vi "myRIO_BRig_Host_endExp_storeFiles__v3.vi"(0 "input_filePath":path) -> ()   [LabVIEW 2014]
panel:
  out "error2":errorcluster
  out "error1":errorcluster
  in  "input_error":errorcluster
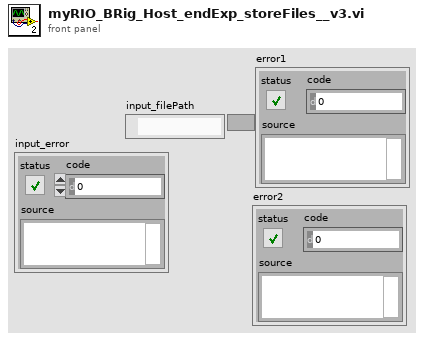
[diagram p1: front panel]
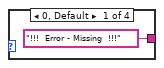
[diagram p2: hidden frame]
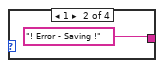
[diagram p3: hidden frame]
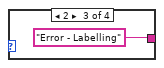
[diagram p4: hidden frame]
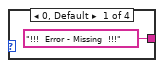
[diagram p5: hidden frame]
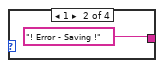
[diagram p6: hidden frame]
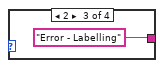
[diagram p7: hidden frame]
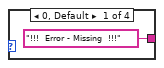
[diagram p8: hidden frame]
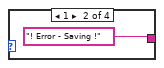
[diagram p9: hidden frame]
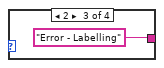
[diagram p10: hidden frame]
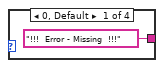
[diagram p11: hidden frame]
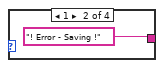
[diagram p12: hidden frame]
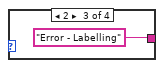
[diagram p13: hidden frame]
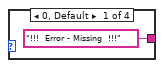
[diagram p14: hidden frame]
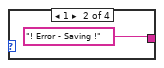
[diagram p15: hidden frame]
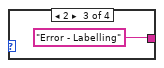
[diagram p16: hidden frame]
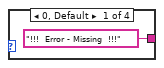
[diagram p17: hidden frame]
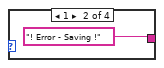
[diagram p18: hidden frame]
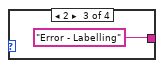
[diagram p19: hidden frame]
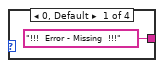
[diagram p20: hidden frame]
diagram:
  w2 = "\r"
  # "Workbooks"
  # "Application"
  # "Is Excel Running?"
  n1 = flat-sequence {
    tunnel: "input_filePath" -> [w358]
    tunnel: "input_error" -> [w355]
    tunnel: [w354] -> w350
    tunnel: [w357] -> w349
    tunnel: [w356] -> w348
    tunnel: [w353] -> w346
    tunnel: w350 -> [w396]
    tunnel: w349 -> [w397]
    tunnel: w348 -> [w360]
    tunnel: [w397] -> w347
    tunnel: w346 -> [w359]
    tunnel: [w396] -> w345
    tunnel: [w392] -> w344
    tunnel: [w391] -> w343
    tunnel: [w387] -> w269
    tunnel: [w386] -> w262
    tunnel: [w383] -> w234
    tunnel: [w380] -> w233
    tunnel: [w379] -> w232
    tunnel: [w378] -> w231
    tunnel: [w372] -> w223
    tunnel: [w371] -> w222
    tunnel: [w367] -> w221
    tunnel: [w366] -> w220
    tunnel: [w362] -> w219
    tunnel: [w361] -> w218
    tunnel: w347 -> [w434]
    tunnel: w345 -> [w430]
    tunnel: w344 -> [w429]
    tunnel: w343 -> [w433]
    tunnel: [w434] -> w342
    tunnel: [w432] -> w341
    tunnel: [w431] -> w340
    tunnel: [w403] -> w339
    tunnel: [w429] -> w338
    tunnel: [w428] -> w270
    tunnel: w269 -> [w428]
    tunnel: [w426] -> w263
    tunnel: w262 -> [w427]
    tunnel: [w425] -> w261
    tunnel: w234 -> [w423]
    tunnel: w233 -> [w422]
    tunnel: w232 -> [w410]
    tunnel: w231 -> [w412]
    tunnel: [w423] -> w225
    tunnel: w223 -> [w421]
    tunnel: w222 -> [w414]
    tunnel: w221 -> [w420]
    tunnel: w220 -> [w416]
    tunnel: w219 -> [w419]
    tunnel: w218 -> [w418]
    tunnel: [w409] -> w212
    tunnel: [w422] -> w206
    tunnel: [w411] -> w200
    tunnel: [w421] -> w194
    tunnel: [w413] -> w188
    tunnel: [w420] -> w182
    tunnel: [w415] -> w176
    tunnel: [w419] -> w170
    tunnel: [w417] -> w164
    tunnel: [w402] -> w163
    tunnel: [w401] -> w153
    tunnel: [w400] -> w145
    tunnel: [w399] -> w139
    tunnel: [w398] -> w134
    tunnel: w342 -> [w471]
    tunnel: w341 -> [w469]
    tunnel: w340 -> [w468]
    tunnel: w339 -> [w443]
    tunnel: w338 -> [w470]
    tunnel: [w471] -> w325
    tunnel: [w470] -> w323
    tunnel: [w469] -> w321
    tunnel: [w468] -> w319
    tunnel: [w467] -> w317
    tunnel: [w462] -> w315
    tunnel: [w464] -> w271
    tunnel: w270 -> [w464]
    tunnel: [w465] -> w264
    tunnel: w263 -> [w465]
    tunnel: w261 -> [w466]
    tunnel: [w466] -> w260
    tunnel: [w463] -> w256
    tunnel: [w459] -> w226
    tunnel: w225 -> [w459]
    tunnel: [w460] -> w213
    tunnel: w212 -> [w460]
    tunnel: [w455] -> w207
    tunnel: w206 -> [w455]
    tunnel: [w456] -> w201
    tunnel: w200 -> [w456]
    tunnel: [w446] -> w195
    tunnel: w194 -> [w446]
    tunnel: [w449] -> w189
    tunnel: w188 -> [w449]
    tunnel: [w445] -> w183
    tunnel: w182 -> [w445]
    tunnel: [w448] -> w177
    tunnel: w176 -> [w448]
    tunnel: [w444] -> w171
    tunnel: w170 -> [w444]
    tunnel: [w447] -> w165
    tunnel: w164 -> [w447]
    tunnel: w163 -> [w461]
    tunnel: [w461] -> w159
    tunnel: [w458] -> w158
    tunnel: w153 -> [w457]
    tunnel: [w457] -> w151
    tunnel: [w454] -> w148
    tunnel: [w453] -> w146
    tunnel: w145 -> [w450]
    tunnel: [w450] -> w140
    tunnel: w139 -> [w451]
    tunnel: [w451] -> w135
    tunnel: w134 -> [w452]
    tunnel: [w452] -> w130
    tunnel: [w442] -> w129
    tunnel: [w441] -> w124
    tunnel: [w440] -> w119
    tunnel: [w439] -> w110
    tunnel: [w438] -> w108
    tunnel: [w437] -> w106
    tunnel: [w436] -> w104
    tunnel: [w435] -> w102
    tunnel: w325 -> [w566]
    tunnel: [w566] -> w324
    tunnel: w323 -> [w565]
    tunnel: [w565] -> w322
    tunnel: w321 -> [w564]
    tunnel: [w564] -> w320
    tunnel: w319 -> [w563]
    tunnel: [w563] -> w318
    tunnel: w317 -> [w561]
    tunnel: [w561] -> w316
    tunnel: w315 -> [w562]
    tunnel: [w562] -> w314
    tunnel: [w557] -> w272
    tunnel: w271 -> [w557]
    tunnel: [w556] -> w265
    tunnel: w264 -> [w556]
    tunnel: w260 -> [w555]
    tunnel: [w555] -> w259
    tunnel: w256 -> [w554]
    tunnel: [w554] -> w255
    tunnel: [w553] -> w227
    tunnel: w226 -> [w553]
    tunnel: [w552] -> w214
    tunnel: w213 -> [w552]
    tunnel: [w551] -> w208
    tunnel: w207 -> [w551]
    tunnel: [w550] -> w202
    tunnel: w201 -> [w550]
    tunnel: [w549] -> w196
    tunnel: w195 -> [w549]
    tunnel: [w548] -> w190
    tunnel: w189 -> [w548]
    tunnel: [w547] -> w184
    tunnel: w183 -> [w547]
    tunnel: [w546] -> w178
    tunnel: w177 -> [w546]
    tunnel: [w545] -> w172
    tunnel: w171 -> [w545]
    tunnel: [w544] -> w166
    tunnel: w165 -> [w544]
    tunnel: [w543] -> w160
    tunnel: w159 -> [w543]
    tunnel: w158 -> [w542]
    tunnel: [w542] -> w154
    tunnel: [w541] -> w152
    tunnel: w151 -> [w541]
    tunnel: w148 -> [w533]
    tunnel: [w540] -> w147
    tunnel: w146 -> [w540]
    tunnel: [w539] -> w141
    tunnel: w140 -> [w539]
    tunnel: [w538] -> w136
    tunnel: w135 -> [w538]
    tunnel: [w537] -> w131
    tunnel: w130 -> [w537]
    tunnel: w129 -> [w536]
    tunnel: [w536] -> w125
    tunnel: w124 -> [w535]
    tunnel: [w535] -> w120
    tunnel: w119 -> [w534]
    tunnel: [w534] -> w115
    tunnel: [w533] -> w111
    tunnel: w110 -> [w532]
    tunnel: [w532] -> w109
    tunnel: w108 -> [w531]
    tunnel: [w531] -> w107
    tunnel: w106 -> [w530]
    tunnel: [w530] -> w105
    tunnel: w104 -> [w529]
    tunnel: [w529] -> w103
    tunnel: w102 -> [w528]
    tunnel: [w528] -> w101
    tunnel: w324 -> [w623]
    tunnel: w322 -> [w622]
    tunnel: w320 -> [w620]
    tunnel: w318 -> [w619]
    tunnel: w316 -> [w621]
    tunnel: w314 -> [w616]
    tunnel: [w623] -> w337
    tunnel: [w622] -> w336
    tunnel: [w621] -> w335
    tunnel: [w603] -> w334
    tunnel: [w618] -> w333
    tunnel: [w617] -> w332
    tunnel: [w615] -> w273
    tunnel: w272 -> [w615]
    tunnel: [w611] -> w266
    tunnel: w265 -> [w613]
    tunnel: w259 -> [w612]
    tunnel: w255 -> [w614]
    tunnel: [w614] -> w254
    tunnel: [w610] -> w251
    tunnel: [w609] -> w228
    tunnel: w227 -> [w609]
    tunnel: [w570] -> w215
    tunnel: w214 -> [w596]
    tunnel: [w608] -> w209
    tunnel: w208 -> [w608]
    tunnel: [w573] -> w203
    tunnel: w202 -> [w593]
    tunnel: [w607] -> w197
    tunnel: w196 -> [w607]
    tunnel: [w576] -> w191
    tunnel: w190 -> [w590]
    tunnel: [w606] -> w185
    tunnel: w184 -> [w606]
    tunnel: [w579] -> w179
    tunnel: w178 -> [w587]
    tunnel: [w605] -> w173
    tunnel: w172 -> [w605]
    tunnel: [w582] -> w167
    tunnel: w166 -> [w597]
    tunnel: w160 -> [w595]
    tunnel: [w604] -> w155
    tunnel: w154 -> [w604]
    tunnel: w152 -> [w592]
    tunnel: w147 -> [w602]
    tunnel: [w581] -> w142
    tunnel: w141 -> [w584]
    tunnel: w136 -> [w586]
    tunnel: w131 -> [w589]
    tunnel: [w601] -> w126
    tunnel: w125 -> [w601]
    tunnel: [w600] -> w121
    tunnel: w120 -> [w600]
    tunnel: [w599] -> w116
    tunnel: w115 -> [w599]
    tunnel: [w598] -> w112
    tunnel: w111 -> [w598]
    tunnel: w109 -> [w594]
    tunnel: w107 -> [w591]
    tunnel: w105 -> [w588]
    tunnel: w103 -> [w585]
    tunnel: w101 -> [w583]
    tunnel: [w580] -> w100
    tunnel: [w578] -> w99
    tunnel: [w577] -> w98
    tunnel: [w575] -> w97
    tunnel: [w574] -> w96
    tunnel: [w572] -> w95
    tunnel: [w571] -> w94
    tunnel: [w569] -> w93
    tunnel: [w568] -> w92
    tunnel: [w567] -> w91
    tunnel: w337 -> [w743]
    tunnel: w336 -> [w741]
    tunnel: w335 -> [w735]
    tunnel: w334 -> [w739]
    tunnel: w333 -> [w742]
    tunnel: w332 -> [w737]
    tunnel: [w743] -> w331
    tunnel: [w741] -> w330
    tunnel: [w740] -> w329
    tunnel: [w727] -> w328
    tunnel: [w742] -> w327
    tunnel: [w737] -> w326
    tunnel: [w733] -> w274
    tunnel: w273 -> [w733]
    tunnel: [w732] -> w267
    tunnel: w266 -> [w732]
    tunnel: [w728] -> w258
    tunnel: w254 -> [w730]
    tunnel: [w729] -> w253
    tunnel: w251 -> [w728]
    tunnel: [w718] -> w229
    tunnel: w228 -> [w718]
    tunnel: [w719] -> w216
    tunnel: w215 -> [w719]
    tunnel: [w711] -> w210
    tunnel: w209 -> [w711]
    tunnel: [w712] -> w204
    tunnel: w203 -> [w712]
    tunnel: [w703] -> w198
    tunnel: w197 -> [w703]
    tunnel: [w704] -> w192
    tunnel: w191 -> [w704]
    tunnel: [w690] -> w186
    tunnel: w185 -> [w690]
    tunnel: [w691] -> w180
    tunnel: w179 -> [w691]
    tunnel: [w684] -> w174
    tunnel: w173 -> [w684]
    tunnel: [w685] -> w168
    tunnel: w167 -> [w685]
    tunnel: [w721] -> w161
    tunnel: [w723] -> w156
    tunnel: w155 -> [w724]
    tunnel: [w715] -> w149
    tunnel: [w692] -> w143
    tunnel: w142 -> [w692]
    tunnel: [w693] -> w137
    tunnel: [w694] -> w132
    tunnel: [w680] -> w127
    tunnel: w126 -> [w682]
    tunnel: [w687] -> w122
    tunnel: w121 -> [w686]
    tunnel: [w700] -> w117
    tunnel: w116 -> [w701]
    tunnel: [w709] -> w113
    tunnel: w112 -> [w708]
    tunnel: w100 -> [w683]
    tunnel: w99 -> [w693]
    tunnel: w98 -> [w689]
    tunnel: w97 -> [w694]
    tunnel: w96 -> [w702]
    tunnel: w95 -> [w715]
    tunnel: w94 -> [w710]
    tunnel: w93 -> [w721]
    tunnel: w92 -> [w717]
    tunnel: w91 -> [w726]
    tunnel: [w725] -> w89
    tunnel: [w716] -> w87
    tunnel: [w707] -> w85
    tunnel: [w699] -> w83
    tunnel: [w688] -> w81
    tunnel: [w681] -> w79
    tunnel: w331 -> [w830]
    tunnel: w330 -> [w835]
    tunnel: w329 -> [w834]
    tunnel: w328 -> [w833]
    tunnel: w327 -> [w832]
    tunnel: w326 -> [w831]
    tunnel: [w830] -> w313
    tunnel: [w835] -> w312
    tunnel: [w834] -> w311
    tunnel: [w833] -> w310
    tunnel: [w832] -> w309
    tunnel: [w831] -> w308
    tunnel: [w829] -> w275
    tunnel: w274 -> [w829]
    tunnel: [w828] -> w268
    tunnel: w267 -> [w828]
    tunnel: w258 -> [w827]
    tunnel: [w827] -> w257
    tunnel: w253 -> [w826]
    tunnel: [w826] -> w252
    tunnel: [w825] -> w230
    tunnel: w229 -> [w825]
    tunnel: [w824] -> w217
    tunnel: w216 -> [w824]
    tunnel: [w823] -> w211
    tunnel: w210 -> [w823]
    tunnel: [w822] -> w205
    tunnel: w204 -> [w822]
    tunnel: [w821] -> w199
    tunnel: w198 -> [w821]
    tunnel: [w820] -> w193
    tunnel: w192 -> [w820]
    tunnel: [w819] -> w187
    tunnel: w186 -> [w819]
    tunnel: [w818] -> w181
    tunnel: w180 -> [w818]
    tunnel: [w817] -> w175
    tunnel: w174 -> [w817]
    tunnel: [w816] -> w169
    tunnel: w168 -> [w816]
    tunnel: [w815] -> w162
    tunnel: w161 -> [w815]
    tunnel: [w814] -> w157
    tunnel: w156 -> [w814]
    tunnel: [w813] -> w150
    tunnel: w149 -> [w813]
    tunnel: [w812] -> w144
    tunnel: w143 -> [w812]
    tunnel: [w811] -> w138
    tunnel: w137 -> [w811]
    tunnel: [w810] -> w133
    tunnel: w132 -> [w810]
    tunnel: [w809] -> w128
    tunnel: w127 -> [w809]
    tunnel: [w808] -> w123
    tunnel: w122 -> [w808]
    tunnel: [w807] -> w118
    tunnel: w117 -> [w807]
    tunnel: [w806] -> w114
    tunnel: w113 -> [w806]
    tunnel: [w805] -> w90
    tunnel: w89 -> [w805]
    tunnel: [w804] -> w88
    tunnel: w87 -> [w804]
    tunnel: [w803] -> w86
    tunnel: w85 -> [w803]
    tunnel: [w802] -> w84
    tunnel: w83 -> [w802]
    tunnel: [w801] -> w82
    tunnel: w81 -> [w801]
    tunnel: [w800] -> w80
    tunnel: w79 -> [w800]
    tunnel: w313 -> [w874]
    tunnel: w312 -> [w882]
    tunnel: w311 -> [w881]
    tunnel: w310 -> [w880]
    tunnel: w309 -> [w879]
    tunnel: w308 -> [w878]
    tunnel: [w874] -> w305
    tunnel: [w882] -> w301
    tunnel: [w881] -> w300
    tunnel: [w880] -> w297
    tunnel: [w879] -> w299
    tunnel: [w878] -> w298
    tunnel: [w870] -> w304
    tunnel: [w869] -> w303
    tunnel: [w868] -> w302
    tunnel: [w867] -> w250
    tunnel: w275 -> [w867]
    tunnel: [w866] -> w248
    tunnel: w268 -> [w866]
    tunnel: w257 -> [w865]
    tunnel: [w865] -> w247
    tunnel: w252 -> [w864]
    tunnel: [w864] -> w249
    tunnel: [w863] -> w224
    tunnel: w230 -> [w863]
    tunnel: [w862] -> w77
    tunnel: w217 -> [w862]
    tunnel: [w861] -> w75
    tunnel: w211 -> [w861]
    tunnel: [w860] -> w73
    tunnel: w205 -> [w860]
    tunnel: [w859] -> w71
    tunnel: w199 -> [w859]
    tunnel: [w858] -> w69
    tunnel: w193 -> [w858]
    tunnel: [w857] -> w67
    tunnel: w187 -> [w857]
    tunnel: [w856] -> w65
    tunnel: w181 -> [w856]
    tunnel: [w855] -> w63
    tunnel: w175 -> [w855]
    tunnel: [w854] -> w61
    tunnel: w169 -> [w854]
    tunnel: [w853] -> w76
    tunnel: w162 -> [w853]
    tunnel: [w852] -> w78
    tunnel: w157 -> [w852]
    tunnel: [w851] -> w72
    tunnel: w150 -> [w851]
    tunnel: [w850] -> w60
    tunnel: w144 -> [w850]
    tunnel: [w849] -> w64
    tunnel: w138 -> [w849]
    tunnel: [w848] -> w68
    tunnel: w133 -> [w848]
    tunnel: [w847] -> w62
    tunnel: w128 -> [w847]
    tunnel: [w846] -> w66
    tunnel: w123 -> [w846]
    tunnel: [w845] -> w70
    tunnel: w118 -> [w845]
    tunnel: [w844] -> w74
    tunnel: w114 -> [w844]
    tunnel: [w843] -> w59
    tunnel: w90 -> [w843]
    tunnel: [w842] -> w58
    tunnel: w88 -> [w842]
    tunnel: [w841] -> w57
    tunnel: w86 -> [w841]
    tunnel: [w840] -> w56
    tunnel: w84 -> [w840]
    tunnel: [w839] -> w55
    tunnel: w82 -> [w839]
    tunnel: [w838] -> w54
    tunnel: w80 -> [w838]
    frame #0 {
      # "Is Excel Running?"
      # "Prepare storage"
      # "get Exp Prefix"
      n2 = call "myRIO_BRig_Host_endExp_getExp.vi"("input_filePath"=w358) -> ("output_expPrefix"=w356:string)  [unwired: 10 in]
      n3 = call "myRIO_BRig_Host_isExcelRunning.vi"() -> ("output_Iexcel"=w357:bool)  [unwired: 11 in]
      n4 = call "myRIO_BRig_Host_endExp_prepareStoreLocation.vi"("input_error"=w355, "input_expPrefix"=w356) -> ("output_error"=w354:errorcluster, "output_folderPath"=w353:string)  [unwired: 8 in]
    }
    frame #1 {
      w363 = "dataTrial" ("input_fileName")
      w368 = "dataMTrig" ("input_fileName")
      w373 = "dataLick" ("input_fileName")
      w377 = "dataLC" ("input_fileName")
      w376 = "dataExp" ("input_fileName")
      w388 = "dataCurrent" ("input_fileName")
      w395 = "dataBlock" ("input_fileName")
      # "original"
      # "storage"
      # "original"
      # "storage"
      # "original"
      # "storage"
      # "original"
      # "storage"
      # "original"
      # "storage"
      # "original"
      # "storage"
      # "original"
      # "storage"
      # "Prepare file paths"
      n5 = call "myRIO_BRig_Host_endExp_filePath__originalLocation.vi"("input_expPrefix"=w360, "input_fileName"=w376) -> ("output_filePath"=w384:string)  [unwired: 9 in]
      n6 = call "myRIO_BRig_Host_endExp_filePath__storeLocation.vi"("input_expPrefix"=w360, "input_fileName"=w376, "input_filePath_storage"=w359) -> ("output_filePath"=w385:string)  [unwired: 8 in]
      n7 = call "myRIO_BRig_Host_endExp_filePath__originalLocation.vi"("input_expPrefix"=w360, "input_fileName"=w388) -> ("output_filePath"=w389:string)  [unwired: 9 in]
      n8 = call "myRIO_BRig_Host_endExp_filePath__originalLocation.vi"("input_expPrefix"=w360, "input_fileName"=w377) -> ("output_filePath"=w381:string)  [unwired: 9 in]
      n9 = call "myRIO_BRig_Host_endExp_filePath__originalLocation.vi"("input_expPrefix"=w360, "input_fileName"=w373) -> ("output_filePath"=w374:string)  [unwired: 9 in]
      n10 = call "myRIO_BRig_Host_endExp_filePath__originalLocation.vi"("input_expPrefix"=w360, "input_fileName"=w368) -> ("output_filePath"=w369:string)  [unwired: 9 in]
      n11 = call "myRIO_BRig_Host_endExp_filePath__originalLocation.vi"("input_expPrefix"=w360, "input_fileName"=w363) -> ("output_filePath"=w364:string)  [unwired: 9 in]
      n12 = call "myRIO_BRig_Host_endExp_filePath__storeLocation.vi"("input_expPrefix"=w360, "input_fileName"=w388, "input_filePath_storage"=w359) -> ("output_filePath"=w390:string)  [unwired: 8 in]
      n13 = call "myRIO_BRig_Host_endExp_filePath__storeLocation.vi"("input_expPrefix"=w360, "input_fileName"=w377, "input_filePath_storage"=w359) -> ("output_filePath"=w382:string)  [unwired: 8 in]
      n14 = call "myRIO_BRig_Host_endExp_filePath__storeLocation.vi"("input_expPrefix"=w360, "input_fileName"=w373, "input_filePath_storage"=w359) -> ("output_filePath"=w375:string)  [unwired: 8 in]
      n15 = call "myRIO_BRig_Host_endExp_filePath__storeLocation.vi"("input_expPrefix"=w360, "input_fileName"=w368, "input_filePath_storage"=w359) -> ("output_filePath"=w370:string)  [unwired: 8 in]
      n16 = call "myRIO_BRig_Host_endExp_filePath__storeLocation.vi"("input_expPrefix"=w360, "input_fileName"=w363, "input_filePath_storage"=w359) -> ("output_filePath"=w365:string)  [unwired: 8 in]
      n17 = call "myRIO_BRig_Host_endExp_filePath__originalLocation.vi"("input_expPrefix"=w360, "input_fileName"=w395) -> ("output_filePath"=w393:string)  [unwired: 9 in]
      n18 = call "myRIO_BRig_Host_endExp_filePath__storeLocation.vi"("input_expPrefix"=w360, "input_fileName"=w395, "input_filePath_storage"=w359) -> ("output_filePath"=w394:string)  [unwired: 8 in]
      n19 = String To Path(string=w385) -> (path=w383:path)
      n20 = String To Path(string=w384) -> (path=w379:path)
      n21 = String To Path(string=w390) -> (path=w387:path)
      n22 = String To Path(string=w389) -> (path=w386:path)
      n23 = String To Path(string=w382) -> (path=w380:path)
      n24 = String To Path(string=w381) -> (path=w378:path)
      n25 = String To Path(string=w375) -> (path=w372:path)
      n26 = String To Path(string=w374) -> (path=w371:path)
      n27 = String To Path(string=w370) -> (path=w367:path)
      n28 = String To Path(string=w369) -> (path=w366:path)
      n29 = String To Path(string=w365) -> (path=w362:path)
      n30 = String To Path(string=w364) -> (path=w361:path)
      n31 = String To Path(string=w394) -> (path=w392:path)
      n32 = String To Path(string=w393) -> (path=w391:path)
    }
    frame #2 {
      # "Check if\noriginal files\nexist"
      n33 = call "myRIO_BRig_generic_pathExists_fast_pathInput.vi"("input_error"=w430, "input_filePath"=w433) -> ("output_error"=w424:errorcluster, "output_Iexist"=w431:bool, "output_filePath"=w432:path)  [unwired: 7 in]
      n34 = call "myRIO_BRig_generic_pathExists_fast_pathInput.vi"("input_error"=w424, "input_filePath"=w427) -> ("output_error"=w408:errorcluster, "output_Iexist"=w425:bool, "output_filePath"=w426:path)  [unwired: 7 in]
      n35 = call "myRIO_BRig_generic_pathExists_fast_pathInput.vi"("input_error"=w408, "input_filePath"=w410) -> ("output_error"=w407:errorcluster, "output_Iexist"=w402:bool, "output_filePath"=w409:path)  [unwired: 7 in]
      n36 = call "myRIO_BRig_generic_pathExists_fast_pathInput.vi"("input_error"=w407, "input_filePath"=w412) -> ("output_error"=w406:errorcluster, "output_Iexist"=w401:bool, "output_filePath"=w411:path)  [unwired: 7 in]
      n37 = call "myRIO_BRig_generic_pathExists_fast_pathInput.vi"("input_error"=w406, "input_filePath"=w414) -> ("output_error"=w405:errorcluster, "output_Iexist"=w398:bool, "output_filePath"=w413:path)  [unwired: 7 in]
      n38 = call "myRIO_BRig_generic_pathExists_fast_pathInput.vi"("input_error"=w405, "input_filePath"=w416) -> ("output_error"=w404:errorcluster, "output_Iexist"=w399:bool, "output_filePath"=w415:path)  [unwired: 7 in]
      n39 = call "myRIO_BRig_generic_pathExists_fast_pathInput.vi"("input_error"=w404, "input_filePath"=w418) -> ("output_error"=w403:errorcluster, "output_Iexist"=w400:bool, "output_filePath"=w417:path)  [unwired: 7 in]
    }
    frame #3 {
      # "If original files exist,\nthen store them"
      n40 = case shown="True" w468 {
        selector: w468 -> [w520 w525]
        tunnel: w469 -> [_ w527]
        tunnel: w470 -> [_ w526]
        tunnel: w443 -> [w521 w524]
        tunnel: [w521 w523] -> w462
        tunnel: [w520 w522] -> w467
        frame False {
        }
        frame True {
          n41 = call "myRIO_BRig_generic_pathMove_pathInput.vi"("input_error"=w524, "input_Ioverwrite"=w525, "input_filePath_target"=w526, "input_filePath_source"=w527) -> ("output_error"=w523:errorcluster, "output_Iexist"=w522:bool)  [unwired: 5 in, 1 out]
        }
      }
      n42 = case shown="True" w466 {
        selector: w466 -> [w512 w517]
        tunnel: w465 -> [_ w519]
        tunnel: w464 -> [_ w518]
        tunnel: w443 -> [w513 w516]
        tunnel: [w513 w515] -> w453
        tunnel: [w512 w514] -> w463
        frame False {
        }
        frame True {
          n43 = call "myRIO_BRig_generic_pathMove_pathInput.vi"("input_error"=w516, "input_Ioverwrite"=w517, "input_filePath_target"=w518, "input_filePath_source"=w519) -> ("output_error"=w515:errorcluster, "output_Iexist"=w514:bool)  [unwired: 5 in, 1 out]
        }
      }
      n44 = case shown="True" w461 {
        selector: w461 -> [w504 w509]
        tunnel: w460 -> [_ w511]
        tunnel: w459 -> [_ w510]
        tunnel: w443 -> [w505 w508]
        tunnel: [w505 w507] -> w439
        tunnel: [w504 w506] -> w458
        frame False {
        }
        frame True {
          n45 = call "myRIO_BRig_generic_pathMove_pathInput.vi"("input_error"=w508, "input_Ioverwrite"=w509, "input_filePath_target"=w510, "input_filePath_source"=w511) -> ("output_error"=w507:errorcluster, "output_Iexist"=w506:bool)  [unwired: 5 in, 1 out]
        }
      }
      n46 = case shown="True" w457 {
        selector: w457 -> [w496 w501]
        tunnel: w456 -> [_ w503]
        tunnel: w455 -> [_ w502]
        tunnel: w443 -> [w497 w500]
        tunnel: [w497 w499] -> w438
        tunnel: [w496 w498] -> w454
        frame False {
        }
        frame True {
          n47 = call "myRIO_BRig_generic_pathMove_pathInput.vi"("input_error"=w500, "input_Ioverwrite"=w501, "input_filePath_target"=w502, "input_filePath_source"=w503) -> ("output_error"=w499:errorcluster, "output_Iexist"=w498:bool)  [unwired: 5 in, 1 out]
        }
      }
      n48 = case shown="True" w452 {
        selector: w452 -> [w488 w493]
        tunnel: w449 -> [_ w495]
        tunnel: w446 -> [_ w494]
        tunnel: w443 -> [w489 w492]
        tunnel: [w489 w491] -> w437
        tunnel: [w488 w490] -> w440
        frame False {
        }
        frame True {
          n49 = call "myRIO_BRig_generic_pathMove_pathInput.vi"("input_error"=w492, "input_Ioverwrite"=w493, "input_filePath_target"=w494, "input_filePath_source"=w495) -> ("output_error"=w491:errorcluster, "output_Iexist"=w490:bool)  [unwired: 5 in, 1 out]
        }
      }
      n50 = case shown="True" w451 {
        selector: w451 -> [w480 w485]
        tunnel: w448 -> [_ w487]
        tunnel: w445 -> [_ w486]
        tunnel: w443 -> [w481 w484]
        tunnel: [w481 w483] -> w436
        tunnel: [w480 w482] -> w441
        frame False {
        }
        frame True {
          n51 = call "myRIO_BRig_generic_pathMove_pathInput.vi"("input_error"=w484, "input_Ioverwrite"=w485, "input_filePath_target"=w486, "input_filePath_source"=w487) -> ("output_error"=w483:errorcluster, "output_Iexist"=w482:bool)  [unwired: 5 in, 1 out]
        }
      }
      n52 = case shown="True" w450 {
        selector: w450 -> [w472 w477]
        tunnel: w447 -> [_ w479]
        tunnel: w444 -> [_ w478]
        tunnel: w443 -> [w473 w476]
        tunnel: [w473 w475] -> w435
        tunnel: [w472 w474] -> w442
        frame False {
        }
        frame True {
          n53 = call "myRIO_BRig_generic_pathMove_pathInput.vi"("input_error"=w476, "input_Ioverwrite"=w477, "input_filePath_target"=w478, "input_filePath_source"=w479) -> ("output_error"=w475:errorcluster, "output_Iexist"=w474:bool)  [unwired: 5 in, 1 out]
        }
      }
    }
    frame #4 {
      # "Add a delay\nin case\nall files\nweren't stored"
      n54 = Select(t=u32 0 ("milliseconds to wait"), s=w561, f=u32 200 ("milliseconds to wait")) -> (s? t:f=w560:u32)
      n55 = Wait (ms)(milliseconds to wait=w560) -> ()  [unwired: 1 out]
    }
    frame #5 {
      # "Re-check\noriginal files"
      n56 = case shown="False" w619 {
        selector: w619 -> [_ w678]
        tunnel: w620 -> [w676 w679]
        tunnel: w616 -> [w675 w677]
        tunnel: [w674 w677] -> w603
        tunnel: [w673 w679] -> w618
        tunnel: [w672 w678] -> w617
        frame False {
          n57 = call "myRIO_BRig_generic_pathExists_fast_pathInput.vi"("input_error"=w675, "input_filePath"=w676) -> ("output_error"=w674:errorcluster, "output_Iexist"=w672:bool, "output_filePath"=w673:path)  [unwired: 7 in]
        }
        frame True {
        }
      }
      n58 = case shown="False" w612 {
        selector: w612 -> [_ w670]
        tunnel: w613 -> [w668 w671]
        tunnel: w602 -> [w667 w669]
        tunnel: [w666 w669] -> w567
        tunnel: [w665 w671] -> w611
        tunnel: [w664 w670] -> w610
        frame False {
          n59 = call "myRIO_BRig_generic_pathExists_fast_pathInput.vi"("input_error"=w667, "input_filePath"=w668) -> ("output_error"=w666:errorcluster, "output_Iexist"=w664:bool, "output_filePath"=w665:path)  [unwired: 7 in]
        }
        frame True {
        }
      }
      n60 = case shown="False" w595 {
        selector: w595 -> [_ w662]
        tunnel: w596 -> [w660 w663]
        tunnel: w594 -> [w659 w661]
        tunnel: [w658 w661] -> w568
        tunnel: [w657 w663] -> w570
        tunnel: [w656 w662] -> w569
        frame False {
          n61 = call "myRIO_BRig_generic_pathExists_fast_pathInput.vi"("input_error"=w659, "input_filePath"=w660) -> ("output_error"=w658:errorcluster, "output_Iexist"=w656:bool, "output_filePath"=w657:path)  [unwired: 7 in]
        }
        frame True {
        }
      }
      n62 = case shown="False" w592 {
        selector: w592 -> [_ w654]
        tunnel: w593 -> [w652 w655]
        tunnel: w591 -> [w651 w653]
        tunnel: [w650 w653] -> w571
        tunnel: [w649 w655] -> w573
        tunnel: [w648 w654] -> w572
        frame False {
          n63 = call "myRIO_BRig_generic_pathExists_fast_pathInput.vi"("input_error"=w651, "input_filePath"=w652) -> ("output_error"=w650:errorcluster, "output_Iexist"=w648:bool, "output_filePath"=w649:path)  [unwired: 7 in]
        }
        frame True {
        }
      }
      n64 = case shown="False" w589 {
        selector: w589 -> [_ w646]
        tunnel: w590 -> [w644 w647]
        tunnel: w588 -> [w643 w645]
        tunnel: [w642 w645] -> w574
        tunnel: [w641 w647] -> w576
        tunnel: [w640 w646] -> w575
        frame False {
          n65 = call "myRIO_BRig_generic_pathExists_fast_pathInput.vi"("input_error"=w643, "input_filePath"=w644) -> ("output_error"=w642:errorcluster, "output_Iexist"=w640:bool, "output_filePath"=w641:path)  [unwired: 7 in]
        }
        frame True {
        }
      }
      n66 = case shown="False" w586 {
        selector: w586 -> [_ w638]
        tunnel: w587 -> [w636 w639]
        tunnel: w585 -> [w635 w637]
        tunnel: [w634 w637] -> w577
        tunnel: [w633 w639] -> w579
        tunnel: [w632 w638] -> w578
        frame False {
          n67 = call "myRIO_BRig_generic_pathExists_fast_pathInput.vi"("input_error"=w635, "input_filePath"=w636) -> ("output_error"=w634:errorcluster, "output_Iexist"=w632:bool, "output_filePath"=w633:path)  [unwired: 7 in]
        }
        frame True {
        }
      }
      n68 = case shown="False" w584 {
        selector: w584 -> [_ w630]
        tunnel: w597 -> [w628 w631]
        tunnel: w583 -> [w627 w629]
        tunnel: [w626 w629] -> w580
        tunnel: [w625 w631] -> w582
        tunnel: [w624 w630] -> w581
        frame False {
          n69 = call "myRIO_BRig_generic_pathExists_fast_pathInput.vi"("input_error"=w627, "input_filePath"=w628) -> ("output_error"=w626:errorcluster, "output_Iexist"=w624:bool, "output_filePath"=w625:path)  [unwired: 7 in]
        }
        frame True {
        }
      }
    }
    frame #6 {
      # "Re-check\nstorage"
      n70 = Not(x=w735) -> (.not. x?=w738:bool)
      n71 = Not(x=w730) -> (.not. x?=w734:bool)
      n72 = Not(x=w701) -> (.not. x?=w705:bool)
      n73 = Not(x=w686) -> (.not. x?=w698:bool)
      n74 = Not(x=w708) -> (.not. x?=w714:bool)
      n75 = Not(x=w682) -> (.not. x?=w695:bool)
      n76 = Not(x=w724) -> (.not. x?=w722:bool)
      n77 = And(x=w738, y=w737) -> (x .and. y?=w736:bool)
      n78 = And(x=w734, y=w728) -> (x .and. y?=w731:bool)
      n79 = And(x=w705, y=w694) -> (x .and. y?=w706:bool)
      n80 = And(x=w698, y=w693) -> (x .and. y?=w697:bool)
      n81 = And(x=w714, y=w715) -> (x .and. y?=w713:bool)
      n82 = And(x=w695, y=w692) -> (x .and. y?=w696:bool)
      n83 = And(x=w722, y=w721) -> (x .and. y?=w720:bool)
      n84 = case shown="True" w736 {
        selector: w736 -> [_ w797]
        tunnel: w742 -> [_ w799]
        tunnel: w741 -> [_ w798]
        tunnel: w739 -> [w793 w796]
        tunnel: [w793 w795] -> w727
        tunnel: [w792 w794] -> w740
        tunnel: w735 -> [w792 _]
        frame False {
        }
        frame True {
          n85 = call "myRIO_BRig_generic_pathMove_pathInput.vi"("input_error"=w796, "input_Ioverwrite"=w797, "input_filePath_target"=w798, "input_filePath_source"=w799) -> ("output_error"=w795:errorcluster, "output_Iexist"=w794:bool)  [unwired: 5 in, 1 out]
        }
      }
      n86 = case shown="True" w731 {
        selector: w731 -> [_ w789]
        tunnel: w732 -> [_ w791]
        tunnel: w733 -> [_ w790]
        tunnel: w726 -> [w785 w788]
        tunnel: [w785 w787] -> w725
        tunnel: [w784 w786] -> w729
        tunnel: w730 -> [w784 _]
        frame False {
        }
        frame True {
          n87 = call "myRIO_BRig_generic_pathMove_pathInput.vi"("input_error"=w788, "input_Ioverwrite"=w789, "input_filePath_target"=w790, "input_filePath_source"=w791) -> ("output_error"=w787:errorcluster, "output_Iexist"=w786:bool)  [unwired: 5 in, 1 out]
        }
      }
      n88 = case shown="True" w720 {
        selector: w720 -> [_ w781]
        tunnel: w719 -> [_ w783]
        tunnel: w718 -> [_ w782]
        tunnel: w717 -> [w777 w780]
        tunnel: [w777 w779] -> w716
        tunnel: [w776 w778] -> w723
        tunnel: w724 -> [w776 _]
        frame False {
        }
        frame True {
          n89 = call "myRIO_BRig_generic_pathMove_pathInput.vi"("input_error"=w780, "input_Ioverwrite"=w781, "input_filePath_target"=w782, "input_filePath_source"=w783) -> ("output_error"=w779:errorcluster, "output_Iexist"=w778:bool)  [unwired: 5 in, 1 out]
        }
      }
      n90 = case shown="True" w713 {
        selector: w713 -> [_ w773]
        tunnel: w712 -> [_ w775]
        tunnel: w711 -> [_ w774]
        tunnel: w710 -> [w769 w772]
        tunnel: [w769 w771] -> w707
        tunnel: [w768 w770] -> w709
        tunnel: w708 -> [w768 _]
        frame False {
        }
        frame True {
          n91 = call "myRIO_BRig_generic_pathMove_pathInput.vi"("input_error"=w772, "input_Ioverwrite"=w773, "input_filePath_target"=w774, "input_filePath_source"=w775) -> ("output_error"=w771:errorcluster, "output_Iexist"=w770:bool)  [unwired: 5 in, 1 out]
        }
      }
      n92 = case shown="True" w706 {
        selector: w706 -> [_ w765]
        tunnel: w704 -> [_ w767]
        tunnel: w703 -> [_ w766]
        tunnel: w702 -> [w761 w764]
        tunnel: [w761 w763] -> w699
        tunnel: [w760 w762] -> w700
        tunnel: w701 -> [w760 _]
        frame False {
        }
        frame True {
          n93 = call "myRIO_BRig_generic_pathMove_pathInput.vi"("input_error"=w764, "input_Ioverwrite"=w765, "input_filePath_target"=w766, "input_filePath_source"=w767) -> ("output_error"=w763:errorcluster, "output_Iexist"=w762:bool)  [unwired: 5 in, 1 out]
        }
      }
      n94 = case shown="True" w697 {
        selector: w697 -> [_ w757]
        tunnel: w691 -> [_ w759]
        tunnel: w690 -> [_ w758]
        tunnel: w689 -> [w753 w756]
        tunnel: [w753 w755] -> w688
        tunnel: [w752 w754] -> w687
        tunnel: w686 -> [w752 _]
        frame False {
        }
        frame True {
          n95 = call "myRIO_BRig_generic_pathMove_pathInput.vi"("input_error"=w756, "input_Ioverwrite"=w757, "input_filePath_target"=w758, "input_filePath_source"=w759) -> ("output_error"=w755:errorcluster, "output_Iexist"=w754:bool)  [unwired: 5 in, 1 out]
        }
      }
      n96 = case shown="True" w696 {
        selector: w696 -> [_ w749]
        tunnel: w685 -> [_ w751]
        tunnel: w684 -> [_ w750]
        tunnel: w683 -> [w745 w748]
        tunnel: [w745 w747] -> w681
        tunnel: [w744 w746] -> w680
        tunnel: w682 -> [w744 _]
        frame False {
        }
        frame True {
          n97 = call "myRIO_BRig_generic_pathMove_pathInput.vi"("input_error"=w748, "input_Ioverwrite"=w749, "input_filePath_target"=w750, "input_filePath_source"=w751) -> ("output_error"=w747:errorcluster, "output_Iexist"=w746:bool)  [unwired: 5 in, 1 out]
        }
      }
    }
    frame #7 {
      # "Check if Excel\nis running"
      n98 = case shown="True" w830 {
        frame False {
        }
        frame True {
          n99 = One Button Dialog(message="!!! Warning !!!  Save all Excel work, then press okay\n(If Excel isn't visible, use Ctrl-Alt-Delete)", button name ("OK")="I have saved any Excel work") -> ()  [unwired: 1 out]
        }
      }
    }
    frame #8 {
      w877 = refnum<k7> refnum  # Excel._Application
      # "Is Excel Running?"
      # "Open Excel via LabView"
      # "Workbooks"
      # "Application"
      n100 = Automation Open(Automation Refnum=w877) -> (Automation Refnum=w876:refnum<k7>, error out=w875:errorcluster)  [unwired: 1 in, 2 out]
      n101 = case shown="False" w874 {
        tunnel: w876 -> [w886 w889]
        tunnel: w875 -> [w885 w888]
        tunnel: [w884 w888] -> w872
        tunnel: [w883 w889] -> w871
        frame False {
          n102 = property class="_Application"(reference=w886, error in=w885, "Visible"=FALSE) -> (reference out=w883:refnum<k7>, error out=w884:errorcluster)
        }
        frame True {
        }
      }
      n103 = property class="_Application"(reference=w871, error in=w872, "DisplayAlerts"=FALSE) -> (reference out=w869:refnum<k7>, error out=w870:errorcluster, "Workbooks"=w868:refnum<k7>)
    }
  }
  n104 = Unbundle By Name(w304) -> ("code"=w307:i32)
  n105 = Equal To 0?(x=w307) -> (x = 0?=w306:bool)
  n106 = case shown="True" w306 {
    tunnel: w305 -> [w908 w1238]
    tunnel: w304 -> [w907 w1237]
    tunnel: w303 -> [w906 w1236]
    tunnel: w302 -> [w905 w1235]
    tunnel: w301 -> [_ w1234]
    tunnel: w300 -> [w903 w1233]
    tunnel: w299 -> [_ w1232]
    tunnel: w298 -> [w902 w1231]
    tunnel: w297 -> [w904 w1226]
    tunnel: [w908 w1175] -> w293
    tunnel: [w907 w1176] -> w294
    tunnel: [w906 w1174] -> w295
    tunnel: [w905 w1173] -> w296
    tunnel: [w904 w924] -> w288
    tunnel: [w902 w1172] -> w282
    tunnel: [_ w1171] -> w283
    tunnel: [w903 w1170] -> w284
    tunnel: w250 -> [_ w1169]
    tunnel: w249 -> [w901 w1168]
    tunnel: w248 -> [_ w1167]
    tunnel: w247 -> [w900 w1166]
    tunnel: [w901 w1150] -> w240
    tunnel: [w900 w1144] -> w238
    tunnel: [_ w1134] -> w239
    tunnel: w224 -> [_ w1132]
    tunnel: w78 -> [w899 w1130]
    tunnel: w77 -> [_ w1128]
    tunnel: w76 -> [w898 w1126]
    tunnel: w75 -> [_ w1124]
    tunnel: w74 -> [w897 w1122]
    tunnel: w73 -> [_ w1120]
    tunnel: w72 -> [w896 w1118]
    tunnel: w71 -> [_ w1116]
    tunnel: w70 -> [w895 w1114]
    tunnel: w69 -> [_ w1112]
    tunnel: w68 -> [w894 w1110]
    tunnel: w67 -> [_ w1108]
    tunnel: w66 -> [w893 w1106]
    tunnel: w65 -> [_ w1104]
    tunnel: w64 -> [w892 w1102]
    tunnel: w63 -> [_ w1100]
    tunnel: w62 -> [w891 w1098]
    tunnel: w61 -> [_ w1096]
    tunnel: w60 -> [w890 w1094]
    tunnel: w59 -> [_ w1093]
    tunnel: w58 -> [_ w1089]
    tunnel: w57 -> [_ w1087]
    tunnel: w56 -> [_ w1085]
    tunnel: w55 -> [_ w1083]
    tunnel: w54 -> [_ w1081]
    tunnel: [w899 w931] -> w7
    tunnel: [_ w930] -> w8
    tunnel: [w898 w929] -> w9
    tunnel: [w897 w920] -> w10
    tunnel: [_ w919] -> w11
    tunnel: [w896 w918] -> w12
    tunnel: [w895 w917] -> w13
    tunnel: [_ w916] -> w14
    tunnel: [w894 w915] -> w15
    tunnel: [w893 w914] -> w16
    tunnel: [_ w913] -> w17
    tunnel: [w892 w912] -> w18
    tunnel: [w891 w911] -> w21
    tunnel: [_ w910] -> w20
    tunnel: [w890 w909] -> w19
    frame False {
    }
    frame True {
      n107 = flat-sequence {
        tunnel: w1238 -> [w1298]
        tunnel: w1237 -> [w1295]
        tunnel: w1236 -> [w1297]
        tunnel: w1235 -> [w1289]
        tunnel: w1234 -> [w1294]
        tunnel: w1233 -> [w1293]
        tunnel: w1232 -> [w1292]
        tunnel: w1231 -> [w1291]
        tunnel: [w1298] -> w1230
        tunnel: [w1297] -> w1229
        tunnel: [w1267] -> w1228
        tunnel: [w1296] -> w1227
        tunnel: w1226 -> [w1296]
        tunnel: [w1266] -> w1225
        tunnel: [w1294] -> w1224
        tunnel: [w1293] -> w1223
        tunnel: [w1292] -> w1222
        tunnel: [w1291] -> w1221
        tunnel: [w1290] -> w1220
        tunnel: w1169 -> [w1286]
        tunnel: w1168 -> [w1285]
        tunnel: w1167 -> [w1288]
        tunnel: w1166 -> [w1287]
        tunnel: [w1286] -> w1161
        tunnel: [w1288] -> w1156
        tunnel: [w1285] -> w1155
        tunnel: [w1287] -> w1149
        tunnel: [w1284] -> w1143
        tunnel: [w1255] -> w1133
        tunnel: w1132 -> [w1255]
        tunnel: [w1254] -> w1131
        tunnel: w1130 -> [w1254]
        tunnel: [w1281] -> w1129
        tunnel: w1128 -> [w1281]
        tunnel: [w1280] -> w1127
        tunnel: w1126 -> [w1280]
        tunnel: [w1251] -> w1125
        tunnel: w1124 -> [w1251]
        tunnel: [w1250] -> w1123
        tunnel: w1122 -> [w1250]
        tunnel: [w1253] -> w1121
        tunnel: w1120 -> [w1253]
        tunnel: [w1252] -> w1119
        tunnel: w1118 -> [w1252]
        tunnel: [w1249] -> w1117
        tunnel: w1116 -> [w1249]
        tunnel: [w1248] -> w1115
        tunnel: w1114 -> [w1248]
        tunnel: [w1279] -> w1113
        tunnel: w1112 -> [w1279]
        tunnel: [w1278] -> w1111
        tunnel: w1110 -> [w1278]
        tunnel: [w1247] -> w1109
        tunnel: w1108 -> [w1247]
        tunnel: [w1246] -> w1107
        tunnel: w1106 -> [w1246]
        tunnel: [w1277] -> w1105
        tunnel: w1104 -> [w1277]
        tunnel: [w1276] -> w1103
        tunnel: w1102 -> [w1276]
        tunnel: [w1245] -> w1101
        tunnel: w1100 -> [w1245]
        tunnel: [w1244] -> w1099
        tunnel: w1098 -> [w1244]
        tunnel: [w1275] -> w1097
        tunnel: w1096 -> [w1275]
        tunnel: [w1274] -> w1095
        tunnel: w1094 -> [w1274]
        tunnel: w1093 -> [w1273]
        tunnel: [w1273] -> w1092
        tunnel: [w1272] -> w1090
        tunnel: w1089 -> [w1272]
        tunnel: [w1271] -> w1088
        tunnel: w1087 -> [w1271]
        tunnel: [w1270] -> w1086
        tunnel: w1085 -> [w1270]
        tunnel: [w1269] -> w1084
        tunnel: w1083 -> [w1269]
        tunnel: [w1268] -> w1082
        tunnel: w1081 -> [w1268]
        tunnel: [w1243] -> w1080
        tunnel: [w1242] -> w1079
        tunnel: [w1241] -> w1078
        tunnel: [w1240] -> w1077
        tunnel: [w1239] -> w1076
        tunnel: w1230 -> [w1428]
        tunnel: w1229 -> [w1431]
        tunnel: w1228 -> [w1430]
        tunnel: w1227 -> [w1415]
        tunnel: w1225 -> [w1429]
        tunnel: w1224 -> [w1432]
        tunnel: w1223 -> [w1433]
        tunnel: w1222 -> [w1435]
        tunnel: w1221 -> [w1434]
        tunnel: w1220 -> [w1410]
        tunnel: [w1435] -> w1219
        tunnel: [w1434] -> w1218
        tunnel: [w1433] -> w1217
        tunnel: [w1432] -> w1216
        tunnel: [w1431] -> w1215
        tunnel: [w1430] -> w1214
        tunnel: [w1429] -> w1213
        tunnel: [w1428] -> w1212
        tunnel: [w1414] -> w1211
        tunnel: [w1412] -> w1210
        tunnel: [w1427] -> w1162
        tunnel: w1161 -> [w1427]
        tunnel: [w1426] -> w1157
        tunnel: w1156 -> [w1426]
        tunnel: w1155 -> [w1425]
        tunnel: [w1425] -> w1154
        tunnel: w1149 -> [w1424]
        tunnel: [w1424] -> w1148
        tunnel: w1143 -> [w1409]
        tunnel: [w1413] -> w1142
        tunnel: [w1411] -> w1141
        tunnel: w1133 -> [w1403]
        tunnel: w1131 -> [w1402]
        tunnel: w1129 -> [w1401]
        tunnel: w1127 -> [w1400]
        tunnel: w1125 -> [w1398]
        tunnel: w1123 -> [w1397]
        tunnel: w1121 -> [w1396]
        tunnel: w1119 -> [w1395]
        tunnel: w1117 -> [w1393]
        tunnel: w1115 -> [w1392]
        tunnel: w1113 -> [w1391]
        tunnel: w1111 -> [w1390]
        tunnel: w1109 -> [w1388]
        tunnel: w1107 -> [w1387]
        tunnel: w1105 -> [w1386]
        tunnel: w1103 -> [w1385]
        tunnel: w1101 -> [w1383]
        tunnel: w1099 -> [w1382]
        tunnel: w1097 -> [w1381]
        tunnel: w1095 -> [w1380]
        tunnel: w1092 -> [w1423]
        tunnel: [w1423] -> w1091
        tunnel: w1090 -> [w1399]
        tunnel: w1088 -> [w1394]
        tunnel: w1086 -> [w1389]
        tunnel: w1084 -> [w1384]
        tunnel: w1082 -> [w1379]
        tunnel: w1080 -> [w1408]
        tunnel: w1079 -> [w1407]
        tunnel: w1078 -> [w1406]
        tunnel: w1077 -> [w1405]
        tunnel: w1076 -> [w1404]
        tunnel: [w1416] -> w1075
        tunnel: [w1403] -> w1071
        tunnel: [w1402] -> w1067
        tunnel: [w1401] -> w1063
        tunnel: [w1400] -> w1059
        tunnel: [w1399] -> w1055
        tunnel: [w1398] -> w1051
        tunnel: [w1397] -> w1047
        tunnel: [w1396] -> w1043
        tunnel: [w1395] -> w1040
        tunnel: [w1394] -> w1036
        tunnel: [w1393] -> w1032
        tunnel: [w1392] -> w1028
        tunnel: [w1391] -> w1024
        tunnel: [w1390] -> w1020
        tunnel: [w1389] -> w1017
        tunnel: [w1388] -> w1013
        tunnel: [w1387] -> w1009
        tunnel: [w1386] -> w1005
        tunnel: [w1385] -> w1002
        tunnel: [w1384] -> w998
        tunnel: [w1383] -> w994
        tunnel: [w1382] -> w990
        tunnel: [w1381] -> w986
        tunnel: [w1380] -> w983
        tunnel: [w1379] -> w979
        tunnel: [w1378] -> w971
        tunnel: [w1377] -> w969
        tunnel: [w1376] -> w967
        tunnel: [w1375] -> w965
        tunnel: [w1374] -> w963
        tunnel: [w1373] -> w961
        tunnel: [w1372] -> w959
        tunnel: [w1371] -> w957
        tunnel: [w1370] -> w955
        tunnel: [w1369] -> w953
        tunnel: w1219 -> [w1498]
        tunnel: w1218 -> [w1499]
        tunnel: w1217 -> [w1509]
        tunnel: w1216 -> [w1508]
        tunnel: w1215 -> [w1507]
        tunnel: w1214 -> [w1506]
        tunnel: w1213 -> [w1505]
        tunnel: w1212 -> [w1504]
        tunnel: w1211 -> [w1503]
        tunnel: w1210 -> [w1502]
        tunnel: [w1501] -> w1209
        tunnel: [w1500] -> w1208
        tunnel: [w1509] -> w1207
        tunnel: [w1508] -> w1206
        tunnel: [w1507] -> w1205
        tunnel: [w1506] -> w1204
        tunnel: [w1505] -> w1203
        tunnel: [w1504] -> w1202
        tunnel: [w1503] -> w1201
        tunnel: [w1502] -> w1200
        tunnel: [w1478] -> w1199
        tunnel: [w1496] -> w1163
        tunnel: w1162 -> [w1496]
        tunnel: [w1490] -> w1158
        tunnel: w1157 -> [w1492]
        tunnel: w1154 -> [w1495]
        tunnel: [w1495] -> w1153
        tunnel: w1148 -> [w1491]
        tunnel: [w1489] -> w1147
        tunnel: w1142 -> [w1494]
        tunnel: w1141 -> [w1493]
        tunnel: [w1494] -> w1138
        tunnel: [w1493] -> w1135
        tunnel: w1091 -> [w1477]
        tunnel: w1075 -> [w1497]
        tunnel: [w1488] -> w1072
        tunnel: w1071 -> [w1488]
        tunnel: [w1487] -> w1068
        tunnel: w1067 -> [w1487]
        tunnel: [w1470] -> w1064
        tunnel: w1063 -> [w1475]
        tunnel: [w1471] -> w1060
        tunnel: w1059 -> [w1474]
        tunnel: [w1472] -> w1056
        tunnel: w1055 -> [w1473]
        tunnel: [w1486] -> w1052
        tunnel: w1051 -> [w1486]
        tunnel: [w1485] -> w1048
        tunnel: w1047 -> [w1485]
        tunnel: [w1464] -> w1044
        tunnel: w1043 -> [w1469]
        tunnel: w1040 -> [w1468]
        tunnel: [w1466] -> w1037
        tunnel: w1036 -> [w1467]
        tunnel: [w1484] -> w1033
        tunnel: w1032 -> [w1484]
        tunnel: [w1483] -> w1029
        tunnel: w1028 -> [w1483]
        tunnel: [w1460] -> w1025
        tunnel: w1024 -> [w1461]
        tunnel: [w1459] -> w1021
        tunnel: w1020 -> [w1462]
        tunnel: w1017 -> [w1463]
        tunnel: [w1482] -> w1014
        tunnel: w1013 -> [w1482]
        tunnel: [w1481] -> w1010
        tunnel: w1009 -> [w1481]
        tunnel: [w1452] -> w1006
        tunnel: w1005 -> [w1457]
        tunnel: w1002 -> [w1456]
        tunnel: [w1454] -> w999
        tunnel: w998 -> [w1455]
        tunnel: [w1480] -> w995
        tunnel: w994 -> [w1480]
        tunnel: [w1479] -> w991
        tunnel: w990 -> [w1479]
        tunnel: [w1446] -> w987
        tunnel: w986 -> [w1451]
        tunnel: w983 -> [w1450]
        tunnel: [w1448] -> w980
        tunnel: w979 -> [w1449]
        tunnel: [w1476] -> w978
        tunnel: [w1465] -> w976
        tunnel: [w1458] -> w975
        tunnel: [w1453] -> w974
        tunnel: [w1447] -> w973
        tunnel: [w1445] -> w972
        tunnel: w971 -> [w1445]
        tunnel: [w1444] -> w970
        tunnel: w969 -> [w1444]
        tunnel: [w1443] -> w968
        tunnel: w967 -> [w1443]
        tunnel: [w1442] -> w966
        tunnel: w965 -> [w1442]
        tunnel: [w1441] -> w964
        tunnel: w963 -> [w1441]
        tunnel: [w1440] -> w962
        tunnel: w961 -> [w1440]
        tunnel: [w1439] -> w960
        tunnel: w959 -> [w1439]
        tunnel: [w1438] -> w958
        tunnel: w957 -> [w1438]
        tunnel: [w1437] -> w956
        tunnel: w955 -> [w1437]
        tunnel: [w1436] -> w954
        tunnel: w953 -> [w1436]
        tunnel: w1209 -> [w1637]
        tunnel: w1208 -> [w1639]
        tunnel: w1207 -> [w1633]
        tunnel: w1206 -> [w1636]
        tunnel: w1205 -> [w1646]
        tunnel: w1204 -> [w1645]
        tunnel: w1203 -> [w1644]
        tunnel: w1202 -> [w1643]
        tunnel: w1201 -> [w1642]
        tunnel: w1200 -> [w1641]
        tunnel: w1199 -> [w1635]
        tunnel: [w1637] -> w1198
        tunnel: [w1639] -> w1197
        tunnel: [w1634] -> w1196
        tunnel: [w1636] -> w1195
        tunnel: [w1646] -> w1194
        tunnel: [w1645] -> w1193
        tunnel: [w1644] -> w1192
        tunnel: [w1643] -> w1191
        tunnel: [w1642] -> w1190
        tunnel: [w1641] -> w1189
        tunnel: [w1623] -> w1188
        tunnel: [w1627] -> w1164
        tunnel: w1163 -> [w1627]
        tunnel: [w1628] -> w1159
        tunnel: w1158 -> [w1628]
        tunnel: w1153 -> [w1625]
        tunnel: [w1624] -> w1152
        tunnel: w1147 -> [w1629]
        tunnel: [w1629] -> w1145
        tunnel: [w1632] -> w1139
        tunnel: w1138 -> [w1632]
        tunnel: [w1631] -> w1136
        tunnel: w1135 -> [w1631]
        tunnel: [w1589] -> w1073
        tunnel: w1072 -> [w1589]
        tunnel: [w1597] -> w1069
        tunnel: w1068 -> [w1601]
        tunnel: [w1592] -> w1065
        tunnel: w1064 -> [w1592]
        tunnel: [w1600] -> w1061
        tunnel: w1060 -> [w1600]
        tunnel: [w1593] -> w1057
        tunnel: w1056 -> [w1594]
        tunnel: [w1590] -> w1053
        tunnel: w1052 -> [w1590]
        tunnel: [w1596] -> w1049
        tunnel: w1048 -> [w1599]
        tunnel: [w1591] -> w1045
        tunnel: w1044 -> [w1591]
        tunnel: [w1598] -> w1041
        tunnel: [w1587] -> w1038
        tunnel: w1037 -> [w1588]
        tunnel: [w1573] -> w1034
        tunnel: w1033 -> [w1573]
        tunnel: [w1570] -> w1030
        tunnel: w1029 -> [w1586]
        tunnel: [w1574] -> w1026
        tunnel: w1025 -> [w1574]
        tunnel: [w1585] -> w1022
        tunnel: w1021 -> [w1585]
        tunnel: [w1571] -> w1018
        tunnel: [w1576] -> w1015
        tunnel: w1014 -> [w1576]
        tunnel: [w1568] -> w1011
        tunnel: w1010 -> [w1584]
        tunnel: [w1577] -> w1007
        tunnel: w1006 -> [w1577]
        tunnel: [w1583] -> w1003
        tunnel: [w1569] -> w1000
        tunnel: w999 -> [w1575]
        tunnel: [w1579] -> w996
        tunnel: w995 -> [w1579]
        tunnel: [w1566] -> w992
        tunnel: w991 -> [w1582]
        tunnel: [w1580] -> w988
        tunnel: w987 -> [w1580]
        tunnel: [w1581] -> w984
        tunnel: [w1567] -> w981
        tunnel: w980 -> [w1578]
        tunnel: w978 -> [w1622]
        tunnel: [w1621] -> w977
        tunnel: w976 -> [w1598]
        tunnel: w975 -> [w1572]
        tunnel: w974 -> [w1583]
        tunnel: w973 -> [w1581]
        tunnel: w972 -> [w1612]
        tunnel: w970 -> [w1595]
        tunnel: w968 -> [w1613]
        tunnel: w966 -> [w1614]
        tunnel: w964 -> [w1615]
        tunnel: w962 -> [w1616]
        tunnel: w960 -> [w1617]
        tunnel: w958 -> [w1618]
        tunnel: w956 -> [w1619]
        tunnel: w954 -> [w1620]
        tunnel: [w1620] -> w951
        tunnel: [w1619] -> w949
        tunnel: [w1618] -> w947
        tunnel: [w1617] -> w945
        tunnel: [w1616] -> w943
        tunnel: [w1615] -> w941
        tunnel: [w1614] -> w939
        tunnel: [w1613] -> w937
        tunnel: [w1595] -> w935
        tunnel: [w1612] -> w933
        tunnel: w1198 -> [w1790]
        tunnel: w1197 -> [w1789]
        tunnel: w1196 -> [w1779]
        tunnel: w1195 -> [w1785]
        tunnel: w1194 -> [w1788]
        tunnel: w1193 -> [w1784]
        tunnel: w1192 -> [w1783]
        tunnel: w1191 -> [w1787]
        tunnel: w1190 -> [w1782]
        tunnel: w1189 -> [w1778]
        tunnel: w1188 -> [w1786]
        tunnel: [w1790] -> w1187
        tunnel: [w1789] -> w1186
        tunnel: [w1779] -> w1185
        tunnel: [w1785] -> w1184
        tunnel: [w1788] -> w1183
        tunnel: [w1709] -> w1182
        tunnel: [w1708] -> w1181
        tunnel: [w1787] -> w1180
        tunnel: [w1781] -> w1179
        tunnel: [w1778] -> w1178
        tunnel: [w1786] -> w1177
        tunnel: [w1770] -> w1165
        tunnel: w1164 -> [w1770]
        tunnel: [w1776] -> w1160
        tunnel: w1159 -> [w1776]
        tunnel: w1152 -> [w1772]
        tunnel: [w1772] -> w1151
        tunnel: [w1775] -> w1146
        tunnel: w1145 -> [w1775]
        tunnel: [w1766] -> w1140
        tunnel: w1139 -> [w1767]
        tunnel: [w1773] -> w1137
        tunnel: w1136 -> [w1773]
        tunnel: [w1729] -> w1074
        tunnel: w1073 -> [w1729]
        tunnel: [w1743] -> w1070
        tunnel: w1069 -> [w1743]
        tunnel: [w1765] -> w1066
        tunnel: w1065 -> [w1765]
        tunnel: [w1764] -> w1062
        tunnel: w1061 -> [w1764]
        tunnel: [w1763] -> w1058
        tunnel: w1057 -> [w1763]
        tunnel: [w1728] -> w1054
        tunnel: w1053 -> [w1728]
        tunnel: [w1740] -> w1050
        tunnel: w1049 -> [w1740]
        tunnel: [w1762] -> w1046
        tunnel: w1045 -> [w1762]
        tunnel: [w1761] -> w1042
        tunnel: w1041 -> [w1761]
        tunnel: [w1760] -> w1039
        tunnel: w1038 -> [w1760]
        tunnel: [w1724] -> w1035
        tunnel: w1034 -> [w1724]
        tunnel: [w1738] -> w1031
        tunnel: w1030 -> [w1738]
        tunnel: [w1759] -> w1027
        tunnel: w1026 -> [w1759]
        tunnel: [w1758] -> w1023
        tunnel: w1022 -> [w1758]
        tunnel: [w1757] -> w1019
        tunnel: w1018 -> [w1757]
        tunnel: [w1723] -> w1016
        tunnel: w1015 -> [w1723]
        tunnel: [w1736] -> w1012
        tunnel: w1011 -> [w1736]
        tunnel: [w1756] -> w1008
        tunnel: w1007 -> [w1756]
        tunnel: [w1755] -> w1004
        tunnel: w1003 -> [w1755]
        tunnel: [w1754] -> w1001
        tunnel: w1000 -> [w1754]
        tunnel: [w1721] -> w997
        tunnel: w996 -> [w1721]
        tunnel: [w1734] -> w993
        tunnel: w992 -> [w1734]
        tunnel: [w1753] -> w989
        tunnel: w988 -> [w1753]
        tunnel: [w1752] -> w985
        tunnel: w984 -> [w1752]
        tunnel: [w1751] -> w982
        tunnel: w981 -> [w1751]
        tunnel: w977 -> [w1750]
        tunnel: [w1703] -> w952
        tunnel: w951 -> [w1720]
        tunnel: [w1735] -> w950
        tunnel: w949 -> [w1735]
        tunnel: [w1704] -> w948
        tunnel: w947 -> [w1722]
        tunnel: [w1737] -> w946
        tunnel: w945 -> [w1737]
        tunnel: [w1705] -> w944
        tunnel: w943 -> [w1725]
        tunnel: [w1739] -> w942
        tunnel: w941 -> [w1739]
        tunnel: [w1706] -> w940
        tunnel: w939 -> [w1726]
        tunnel: [w1741] -> w938
        tunnel: w937 -> [w1741]
        tunnel: [w1707] -> w936
        tunnel: w935 -> [w1727]
        tunnel: [w1744] -> w934
        tunnel: w933 -> [w1744]
        tunnel: [w1750] -> w932
        tunnel: w1187 -> [w1941]
        tunnel: w1186 -> [w1940]
        tunnel: w1185 -> [w1939]
        tunnel: w1184 -> [w1938]
        tunnel: w1183 -> [w1937]
        tunnel: w1182 -> [w1936]
        tunnel: w1181 -> [w1935]
        tunnel: w1180 -> [w1934]
        tunnel: w1179 -> [w1932]
        tunnel: w1178 -> [w1930]
        tunnel: w1177 -> [w1929]
        tunnel: [w1941] -> _
        tunnel: [w1940] -> w1172
        tunnel: [w1939] -> w1170
        tunnel: [w1938] -> _
        tunnel: [w1937] -> w1174
        tunnel: [w1936] -> w1173
        tunnel: [w1935] -> w1176
        tunnel: [w1934] -> w1175
        tunnel: [w1932] -> _
        tunnel: [w1931] -> w1171
        tunnel: [w1900] -> w925
        tunnel: [w1928] -> _
        tunnel: w1165 -> [w1928]
        tunnel: [w1927] -> _
        tunnel: w1160 -> [w1927]
        tunnel: w1151 -> [w1926]
        tunnel: [w1926] -> w1150
        tunnel: [w1925] -> w1144
        tunnel: w1146 -> [w1925]
        tunnel: [w1922] -> _
        tunnel: w1140 -> [w1922]
        tunnel: [w1921] -> w1134
        tunnel: w1137 -> [w1923]
        tunnel: [w1920] -> _
        tunnel: w1074 -> [w1920]
        tunnel: [w1919] -> w931
        tunnel: w1070 -> [w1919]
        tunnel: [w1918] -> _
        tunnel: w1066 -> [w1918]
        tunnel: [w1917] -> w929
        tunnel: w1062 -> [w1917]
        tunnel: [w1876] -> w928
        tunnel: w1058 -> [w1878]
        tunnel: [w1916] -> _
        tunnel: w1054 -> [w1916]
        tunnel: [w1915] -> w920
        tunnel: w1050 -> [w1915]
        tunnel: [w1914] -> _
        tunnel: w1046 -> [w1914]
        tunnel: [w1913] -> w918
        tunnel: w1042 -> [w1913]
        tunnel: [w1874] -> w927
        tunnel: w1039 -> [w1879]
        tunnel: [w1912] -> _
        tunnel: w1035 -> [w1912]
        tunnel: [w1911] -> w917
        tunnel: w1031 -> [w1911]
        tunnel: [w1910] -> _
        tunnel: w1027 -> [w1910]
        tunnel: [w1909] -> w915
        tunnel: w1023 -> [w1909]
        tunnel: [w1872] -> w923
        tunnel: w1019 -> [w1880]
        tunnel: [w1908] -> _
        tunnel: w1016 -> [w1908]
        tunnel: [w1907] -> w914
        tunnel: w1012 -> [w1907]
        tunnel: [w1906] -> _
        tunnel: w1008 -> [w1906]
        tunnel: [w1905] -> w912
        tunnel: w1004 -> [w1905]
        tunnel: [w1870] -> w922
        tunnel: w1001 -> [w1881]
        tunnel: [w1904] -> _
        tunnel: w997 -> [w1904]
        tunnel: [w1903] -> w911
        tunnel: w993 -> [w1903]
        tunnel: [w1902] -> _
        tunnel: w989 -> [w1902]
        tunnel: [w1901] -> w909
        tunnel: w985 -> [w1901]
        tunnel: [w1868] -> w921
        tunnel: w982 -> [w1882]
        tunnel: [w1883] -> _
        tunnel: w952 -> [w1883]
        tunnel: [w1869] -> w910
        tunnel: w950 -> [w1888]
        tunnel: [w1884] -> _
        tunnel: w948 -> [w1884]
        tunnel: [w1871] -> w913
        tunnel: w946 -> [w1889]
        tunnel: [w1885] -> _
        tunnel: w944 -> [w1885]
        tunnel: [w1873] -> w916
        tunnel: w942 -> [w1890]
        tunnel: [w1886] -> _
        tunnel: w940 -> [w1886]
        tunnel: [w1875] -> w919
        tunnel: w938 -> [w1891]
        tunnel: [w1887] -> _
        tunnel: w936 -> [w1887]
        tunnel: [w1877] -> w930
        tunnel: w934 -> [w1892]
        tunnel: w932 -> [w1899]
        tunnel: [w1898] -> w926
        frame #0 {
          # "Use Excel\nto add\nheaders"
          n108 = case shown="True" w1293 {
            selector: w1293 -> [_ w1367]
            tunnel: w1294 -> [_ w1366]
            tunnel: w1289 -> [w1360 w1365]
            tunnel: w1295 -> [w1359 w1364]
            tunnel: [w1359 w1362] -> w1282
            tunnel: [w1360 w1363] -> w1283
            tunnel: [_ w1361] -> w1290
            frame False {
            }
            frame True {
              n109 = call "myRIO_BRig_Host_formatData_getHeaders_dataBlock.vi"() -> ("output_stringArray_dataBlock"=w1368:string[])  [unwired: 11 in]
              n110 = call "myRIO_BRig_Host_formatData_test3_p2.vi"("input_headers"=w1368, "input_error"=w1364, "input_Iexist"=w1367, "input_filePath"=w1366, "input_hdl_Workbooks"=w1365) -> ("output_error"=w1362:errorcluster, "output_newFilePath"=w1361:path, "output_hdl_Worksbooks"=w1363:refnum<k7>)  [unwired: 4 in]
            }
          }
          n111 = case shown="True" w1285 {
            selector: w1285 -> [_ w1357]
            tunnel: w1286 -> [_ w1356]
            tunnel: w1283 -> [w1350 w1355]
            tunnel: w1282 -> [w1349 w1354]
            tunnel: [w1349 w1352] -> w1264
            tunnel: [w1350 w1353] -> w1265
            tunnel: [_ w1351] -> w1284
            frame False {
            }
            frame True {
              n112 = call "myRIO_BRig_Host_formatData_getHeaders_dataCurrent.vi"() -> ("output_stringArray_dataCurrent"=w1358:string[])  [unwired: 11 in]
              n113 = call "myRIO_BRig_Host_formatData_test3_p2.vi"("input_headers"=w1358, "input_error"=w1354, "input_Iexist"=w1357, "input_filePath"=w1356, "input_hdl_Workbooks"=w1355) -> ("output_error"=w1352:errorcluster, "output_newFilePath"=w1351:path, "output_hdl_Worksbooks"=w1353:refnum<k7>)  [unwired: 4 in]
            }
          }
          n114 = case shown="True" w1254 {
            selector: w1254 -> [_ w1347]
            tunnel: w1255 -> [_ w1346]
            tunnel: w1265 -> [w1340 w1345]
            tunnel: w1264 -> [w1339 w1344]
            tunnel: [w1339 w1342] -> w1262
            tunnel: [w1340 w1343] -> w1263
            tunnel: [_ w1341] -> w1243
            frame False {
            }
            frame True {
              n115 = call "myRIO_BRig_Host_formatData_getHeaders_dataExp.vi"() -> ("output_stringArray_dataExp"=w1348:string[])  [unwired: 11 in]
              n116 = call "myRIO_BRig_Host_formatData_test3_p2.vi"("input_headers"=w1348, "input_error"=w1344, "input_Iexist"=w1347, "input_filePath"=w1346, "input_hdl_Workbooks"=w1345) -> ("output_error"=w1342:errorcluster, "output_newFilePath"=w1341:path, "output_hdl_Worksbooks"=w1343:refnum<k7>)  [unwired: 4 in]
            }
          }
          n117 = case shown="True" w1250 {
            selector: w1250 -> [_ w1337]
            tunnel: w1251 -> [_ w1336]
            tunnel: w1263 -> [w1330 w1335]
            tunnel: w1262 -> [w1329 w1334]
            tunnel: [w1329 w1332] -> w1260
            tunnel: [w1330 w1333] -> w1261
            tunnel: [_ w1331] -> w1242
            frame False {
            }
            frame True {
              n118 = call "myRIO_BRig_Host_formatData_getHeaders_dataLC.vi"() -> ("output_stringArray_dataLC"=w1338:string[])  [unwired: 11 in]
              n119 = call "myRIO_BRig_Host_formatData_test3_p2.vi"("input_headers"=w1338, "input_error"=w1334, "input_Iexist"=w1337, "input_filePath"=w1336, "input_hdl_Workbooks"=w1335) -> ("output_error"=w1332:errorcluster, "output_newFilePath"=w1331:path, "output_hdl_Worksbooks"=w1333:refnum<k7>)  [unwired: 4 in]
            }
          }
          n120 = case shown="True" w1248 {
            selector: w1248 -> [_ w1327]
            tunnel: w1249 -> [_ w1326]
            tunnel: w1261 -> [w1320 w1325]
            tunnel: w1260 -> [w1319 w1324]
            tunnel: [w1319 w1322] -> w1258
            tunnel: [w1320 w1323] -> w1259
            tunnel: [_ w1321] -> w1241
            frame False {
            }
            frame True {
              n121 = call "myRIO_BRig_Host_formatData_getHeaders_dataLick.vi"() -> ("output_stringArray_dataLick"=w1328:string[])  [unwired: 11 in]
              n122 = call "myRIO_BRig_Host_formatData_test3_p2.vi"("input_headers"=w1328, "input_error"=w1324, "input_Iexist"=w1327, "input_filePath"=w1326, "input_hdl_Workbooks"=w1325) -> ("output_error"=w1322:errorcluster, "output_newFilePath"=w1321:path, "output_hdl_Worksbooks"=w1323:refnum<k7>)  [unwired: 4 in]
            }
          }
          n123 = case shown="True" w1246 {
            selector: w1246 -> [_ w1317]
            tunnel: w1247 -> [_ w1316]
            tunnel: w1259 -> [w1310 w1315]
            tunnel: w1258 -> [w1309 w1314]
            tunnel: [w1309 w1312] -> w1256
            tunnel: [w1310 w1313] -> w1257
            tunnel: [_ w1311] -> w1240
            frame False {
            }
            frame True {
              n124 = call "myRIO_BRig_Host_formatData_getHeaders_dataMTrig.vi"() -> ("output_stringArray_dataMTrig"=w1318:string[])  [unwired: 11 in]
              n125 = call "myRIO_BRig_Host_formatData_test3_p2.vi"("input_headers"=w1318, "input_error"=w1314, "input_Iexist"=w1317, "input_filePath"=w1316, "input_hdl_Workbooks"=w1315) -> ("output_error"=w1312:errorcluster, "output_newFilePath"=w1311:path, "output_hdl_Worksbooks"=w1313:refnum<k7>)  [unwired: 4 in]
            }
          }
          n126 = case shown="True" w1244 {
            selector: w1244 -> [_ w1307]
            tunnel: w1245 -> [_ w1306]
            tunnel: w1257 -> [w1300 w1305]
            tunnel: w1256 -> [w1299 w1304]
            tunnel: [w1299 w1302] -> w1266
            tunnel: [w1300 w1303] -> w1267
            tunnel: [_ w1301] -> w1239
            frame False {
            }
            frame True {
              n127 = call "myRIO_BRig_Host_formatData_getHeaders_dataTrial.vi"() -> ("output_stringArray_dataTrial"=w1308:string[])  [unwired: 11 in]
              n128 = call "myRIO_BRig_Host_formatData_test3_p2.vi"("input_headers"=w1308, "input_error"=w1304, "input_Iexist"=w1307, "input_filePath"=w1306, "input_hdl_Workbooks"=w1305) -> ("output_error"=w1302:errorcluster, "output_newFilePath"=w1301:path, "output_hdl_Worksbooks"=w1303:refnum<k7>)  [unwired: 4 in]
            }
          }
        }
        frame #1 {
          # "Check if\nfile was\ncreated"
          n129 = call "myRIO_BRig_generic_pathExists_fast_pathInput.vi"("input_error"=w1415, "input_filePath"=w1410) -> ("output_error"=w1422:errorcluster, "output_Iexist"=w1412:bool, "output_filePath"=w1414:path)  [unwired: 7 in]
          n130 = call "myRIO_BRig_generic_pathExists_fast_pathInput.vi"("input_error"=w1422, "input_filePath"=w1409) -> ("output_error"=w1421:errorcluster, "output_Iexist"=w1411:bool, "output_filePath"=w1413:path)  [unwired: 7 in]
          n131 = call "myRIO_BRig_generic_pathExists_fast_pathInput.vi"("input_error"=w1421, "input_filePath"=w1408) -> ("output_error"=w1420:errorcluster, "output_Iexist"=w1378:bool, "output_filePath"=w1377:path)  [unwired: 7 in]
          n132 = call "myRIO_BRig_generic_pathExists_fast_pathInput.vi"("input_error"=w1420, "input_filePath"=w1407) -> ("output_error"=w1419:errorcluster, "output_Iexist"=w1376:bool, "output_filePath"=w1375:path)  [unwired: 7 in]
          n133 = call "myRIO_BRig_generic_pathExists_fast_pathInput.vi"("input_error"=w1419, "input_filePath"=w1406) -> ("output_error"=w1418:errorcluster, "output_Iexist"=w1374:bool, "output_filePath"=w1373:path)  [unwired: 7 in]
          n134 = call "myRIO_BRig_generic_pathExists_fast_pathInput.vi"("input_error"=w1418, "input_filePath"=w1405) -> ("output_error"=w1417:errorcluster, "output_Iexist"=w1372:bool, "output_filePath"=w1371:path)  [unwired: 7 in]
          n135 = call "myRIO_BRig_generic_pathExists_fast_pathInput.vi"("input_error"=w1417, "input_filePath"=w1404) -> ("output_error"=w1416:errorcluster, "output_Iexist"=w1370:bool, "output_filePath"=w1369:path)  [unwired: 7 in]
        }
        frame #2 {
          # "Re-check\noriginal files"
          n136 = case shown="False" w1499 {
            selector: w1499 -> [_ w1564]
            tunnel: w1498 -> [w1562 w1565]
            tunnel: w1497 -> [w1561 w1563]
            tunnel: [w1560 w1563] -> w1478
            tunnel: [w1559 w1565] -> w1501
            tunnel: [w1558 w1564] -> w1500
            frame False {
              n137 = call "myRIO_BRig_generic_pathExists_fast_pathInput.vi"("input_error"=w1561, "input_filePath"=w1562) -> ("output_error"=w1560:errorcluster, "output_Iexist"=w1558:bool, "output_filePath"=w1559:path)  [unwired: 7 in]
            }
            frame True {
            }
          }
          n138 = case shown="False" w1491 {
            selector: w1491 -> [_ w1556]
            tunnel: w1492 -> [w1554 w1557]
            tunnel: w1477 -> [w1553 w1555]
            tunnel: [w1552 w1555] -> w1476
            tunnel: [w1551 w1557] -> w1490
            tunnel: [w1550 w1556] -> w1489
            frame False {
              n139 = call "myRIO_BRig_generic_pathExists_fast_pathInput.vi"("input_error"=w1553, "input_filePath"=w1554) -> ("output_error"=w1552:errorcluster, "output_Iexist"=w1550:bool, "output_filePath"=w1551:path)  [unwired: 7 in]
            }
            frame True {
            }
          }
          n140 = case shown="False" w1474 {
            selector: w1474 -> [_ w1548]
            tunnel: w1475 -> [w1546 w1549]
            tunnel: w1473 -> [w1545 w1547]
            tunnel: [w1544 w1547] -> w1472
            tunnel: [w1543 w1549] -> w1470
            tunnel: [w1542 w1548] -> w1471
            frame False {
              n141 = call "myRIO_BRig_generic_pathExists_fast_pathInput.vi"("input_error"=w1545, "input_filePath"=w1546) -> ("output_error"=w1544:errorcluster, "output_Iexist"=w1542:bool, "output_filePath"=w1543:path)  [unwired: 7 in]
            }
            frame True {
            }
          }
          n142 = case shown="False" w1468 {
            selector: w1468 -> [_ w1540]
            tunnel: w1469 -> [w1538 w1541]
            tunnel: w1467 -> [w1537 w1539]
            tunnel: [w1536 w1539] -> w1466
            tunnel: [w1535 w1541] -> w1464
            tunnel: [w1534 w1540] -> w1465
            frame False {
              n143 = call "myRIO_BRig_generic_pathExists_fast_pathInput.vi"("input_error"=w1537, "input_filePath"=w1538) -> ("output_error"=w1536:errorcluster, "output_Iexist"=w1534:bool, "output_filePath"=w1535:path)  [unwired: 7 in]
            }
            frame True {
            }
          }
          n144 = case shown="False" w1462 {
            selector: w1462 -> [_ w1532]
            tunnel: w1461 -> [w1530 w1533]
            tunnel: w1463 -> [w1529 w1531]
            tunnel: [w1528 w1531] -> w1458
            tunnel: [w1527 w1533] -> w1460
            tunnel: [w1526 w1532] -> w1459
            frame False {
              n145 = call "myRIO_BRig_generic_pathExists_fast_pathInput.vi"("input_error"=w1529, "input_filePath"=w1530) -> ("output_error"=w1528:errorcluster, "output_Iexist"=w1526:bool, "output_filePath"=w1527:path)  [unwired: 7 in]
            }
            frame True {
            }
          }
          n146 = case shown="False" w1456 {
            selector: w1456 -> [_ w1524]
            tunnel: w1457 -> [w1522 w1525]
            tunnel: w1455 -> [w1521 w1523]
            tunnel: [w1520 w1523] -> w1454
            tunnel: [w1519 w1525] -> w1452
            tunnel: [w1518 w1524] -> w1453
            frame False {
              n147 = call "myRIO_BRig_generic_pathExists_fast_pathInput.vi"("input_error"=w1521, "input_filePath"=w1522) -> ("output_error"=w1520:errorcluster, "output_Iexist"=w1518:bool, "output_filePath"=w1519:path)  [unwired: 7 in]
            }
            frame True {
            }
          }
          n148 = case shown="False" w1450 {
            selector: w1450 -> [_ w1516]
            tunnel: w1451 -> [w1514 w1517]
            tunnel: w1449 -> [w1513 w1515]
            tunnel: [w1512 w1515] -> w1448
            tunnel: [w1511 w1517] -> w1446
            tunnel: [w1510 w1516] -> w1447
            frame False {
              n149 = call "myRIO_BRig_generic_pathExists_fast_pathInput.vi"("input_error"=w1513, "input_filePath"=w1514) -> ("output_error"=w1512:errorcluster, "output_Iexist"=w1510:bool, "output_filePath"=w1511:path)  [unwired: 7 in]
            }
            frame True {
            }
          }
        }
        frame #3 {
          # "Re-check\nstorage"
          n150 = Not(x=w1633) -> (.not. x?=w1640:bool)
          n151 = Not(x=w1601) -> (.not. x?=w1611:bool)
          n152 = Not(x=w1625) -> (.not. x?=w1630:bool)
          n153 = Not(x=w1599) -> (.not. x?=w1609:bool)
          n154 = Not(x=w1586) -> (.not. x?=w1607:bool)
          n155 = Not(x=w1584) -> (.not. x?=w1605:bool)
          n156 = Not(x=w1582) -> (.not. x?=w1603:bool)
          n157 = And(x=w1640, y=w1639) -> (x .and. y?=w1638:bool)
          n158 = And(x=w1611, y=w1600) -> (x .and. y?=w1610:bool)
          n159 = And(x=w1630, y=w1629) -> (x .and. y?=w1626:bool)
          n160 = And(x=w1609, y=w1598) -> (x .and. y?=w1608:bool)
          n161 = And(x=w1607, y=w1585) -> (x .and. y?=w1606:bool)
          n162 = And(x=w1605, y=w1583) -> (x .and. y?=w1604:bool)
          n163 = And(x=w1603, y=w1581) -> (x .and. y?=w1602:bool)
          n164 = case shown="True" w1638 {
            selector: w1638 -> [_ w1700]
            tunnel: w1637 -> [_ w1702]
            tunnel: w1636 -> [_ w1701]
            tunnel: w1635 -> [w1696 w1699]
            tunnel: [w1696 w1698] -> w1623
            tunnel: [w1695 w1697] -> w1634
            tunnel: w1633 -> [w1695 _]
            frame False {
            }
            frame True {
              n165 = call "myRIO_BRig_generic_pathMove_pathInput.vi"("input_error"=w1699, "input_Ioverwrite"=w1700, "input_filePath_target"=w1701, "input_filePath_source"=w1702) -> ("output_error"=w1698:errorcluster, "output_Iexist"=w1697:bool)  [unwired: 5 in, 1 out]
            }
          }
          n166 = case shown="True" w1610 {
            selector: w1610 -> [_ w1684]
            tunnel: w1592 -> [_ w1686]
            tunnel: w1589 -> [_ w1685]
            tunnel: w1594 -> [w1680 w1683]
            tunnel: [w1680 w1682] -> w1593
            tunnel: [w1679 w1681] -> w1597
            tunnel: w1601 -> [w1679 _]
            frame False {
            }
            frame True {
              n167 = call "myRIO_BRig_generic_pathMove_pathInput.vi"("input_error"=w1683, "input_Ioverwrite"=w1684, "input_filePath_target"=w1685, "input_filePath_source"=w1686) -> ("output_error"=w1682:errorcluster, "output_Iexist"=w1681:bool)  [unwired: 5 in, 1 out]
            }
          }
          n168 = case shown="True" w1626 {
            selector: w1626 -> [_ w1692]
            tunnel: w1628 -> [_ w1694]
            tunnel: w1627 -> [_ w1693]
            tunnel: w1622 -> [w1688 w1691]
            tunnel: [w1688 w1690] -> w1621
            tunnel: [w1687 w1689] -> w1624
            tunnel: w1625 -> [w1687 _]
            frame False {
            }
            frame True {
              n169 = call "myRIO_BRig_generic_pathMove_pathInput.vi"("input_error"=w1691, "input_Ioverwrite"=w1692, "input_filePath_target"=w1693, "input_filePath_source"=w1694) -> ("output_error"=w1690:errorcluster, "output_Iexist"=w1689:bool)  [unwired: 5 in, 1 out]
            }
          }
          n170 = case shown="True" w1608 {
            selector: w1608 -> [_ w1676]
            tunnel: w1591 -> [_ w1678]
            tunnel: w1590 -> [_ w1677]
            tunnel: w1588 -> [w1672 w1675]
            tunnel: [w1672 w1674] -> w1587
            tunnel: [w1671 w1673] -> w1596
            tunnel: w1599 -> [w1671 _]
            frame False {
            }
            frame True {
              n171 = call "myRIO_BRig_generic_pathMove_pathInput.vi"("input_error"=w1675, "input_Ioverwrite"=w1676, "input_filePath_target"=w1677, "input_filePath_source"=w1678) -> ("output_error"=w1674:errorcluster, "output_Iexist"=w1673:bool)  [unwired: 5 in, 1 out]
            }
          }
          n172 = case shown="True" w1606 {
            selector: w1606 -> [_ w1668]
            tunnel: w1574 -> [_ w1670]
            tunnel: w1573 -> [_ w1669]
            tunnel: w1572 -> [w1664 w1667]
            tunnel: [w1664 w1666] -> w1571
            tunnel: [w1663 w1665] -> w1570
            tunnel: w1586 -> [w1663 _]
            frame False {
            }
            frame True {
              n173 = call "myRIO_BRig_generic_pathMove_pathInput.vi"("input_error"=w1667, "input_Ioverwrite"=w1668, "input_filePath_target"=w1669, "input_filePath_source"=w1670) -> ("output_error"=w1666:errorcluster, "output_Iexist"=w1665:bool)  [unwired: 5 in, 1 out]
            }
          }
          n174 = case shown="True" w1604 {
            selector: w1604 -> [_ w1660]
            tunnel: w1577 -> [_ w1662]
            tunnel: w1576 -> [_ w1661]
            tunnel: w1575 -> [w1656 w1659]
            tunnel: [w1656 w1658] -> w1569
            tunnel: [w1655 w1657] -> w1568
            tunnel: w1584 -> [w1655 _]
            frame False {
            }
            frame True {
              n175 = call "myRIO_BRig_generic_pathMove_pathInput.vi"("input_error"=w1659, "input_Ioverwrite"=w1660, "input_filePath_target"=w1661, "input_filePath_source"=w1662) -> ("output_error"=w1658:errorcluster, "output_Iexist"=w1657:bool)  [unwired: 5 in, 1 out]
            }
          }
          n176 = case shown="True" w1602 {
            selector: w1602 -> [_ w1652]
            tunnel: w1580 -> [_ w1654]
            tunnel: w1579 -> [_ w1653]
            tunnel: w1578 -> [w1648 w1651]
            tunnel: [w1648 w1650] -> w1567
            tunnel: [w1647 w1649] -> w1566
            tunnel: w1582 -> [w1647 _]
            frame False {
            }
            frame True {
              n177 = call "myRIO_BRig_generic_pathMove_pathInput.vi"("input_error"=w1651, "input_Ioverwrite"=w1652, "input_filePath_target"=w1653, "input_filePath_source"=w1654) -> ("output_error"=w1650:errorcluster, "output_Iexist"=w1649:bool)  [unwired: 5 in, 1 out]
            }
          }
          n178 = call "myRIO_BRig_Host_formatData_getHeaders_dataCurrent.vi"() -> ()  [unwired: 11 in, 1 out]
          n179 = call "myRIO_BRig_Host_formatData_getHeaders_dataExp.vi"() -> ()  [unwired: 11 in, 1 out]
          n180 = call "myRIO_BRig_Host_formatData_getHeaders_dataLC.vi"() -> ()  [unwired: 11 in, 1 out]
          n181 = call "myRIO_BRig_Host_formatData_getHeaders_dataLick.vi"() -> ()  [unwired: 11 in, 1 out]
        }
        frame #4 {
          # "Re-check\nlabel"
          n182 = Not(x=w1735) -> (.not. x?=w1745:bool)
          n183 = Not(x=w1737) -> (.not. x?=w1746:bool)
          n184 = And(x=w1745, y=w1734) -> (x .and. y?=w1733:bool)
          n185 = And(x=w1746, y=w1736) -> (x .and. y?=w1732:bool)
          n186 = Not(x=w1778) -> (.not. x?=w1777:bool)
          n187 = Not(x=w1739) -> (.not. x?=w1747:bool)
          n188 = Not(x=w1741) -> (.not. x?=w1748:bool)
          n189 = And(x=w1777, y=w1779) -> (x .and. y?=w1780:bool)
          n190 = Not(x=w1773) -> (.not. x?=w1774:bool)
          n191 = And(x=w1747, y=w1738) -> (x .and. y?=w1731:bool)
          n192 = Not(x=w1744) -> (.not. x?=w1749:bool)
          n193 = And(x=w1748, y=w1740) -> (x .and. y?=w1730:bool)
          n194 = And(x=w1774, y=w1772) -> (x .and. y?=w1771:bool)
          n195 = And(x=w1749, y=w1743) -> (x .and. y?=w1742:bool)
          n196 = case shown="True" w1780 {
            selector: w1780 -> [_ w1866]
            tunnel: w1785 -> [_ w1865]
            tunnel: w1784 -> [w1859 w1864]
            tunnel: w1783 -> [w1858 w1863]
            tunnel: [w1858 w1861] -> w1768
            tunnel: [w1859 w1862] -> w1769
            tunnel: [w1857 w1860] -> w1781
            tunnel: w1782 -> [w1857 _]
            frame False {
            }
            frame True {
              n197 = call "myRIO_BRig_Host_formatData_getHeaders_dataBlock.vi"() -> ("output_stringArray_dataBlock"=w1867:string[])  [unwired: 11 in]
              n198 = call "myRIO_BRig_Host_formatData_test3_p2.vi"("input_headers"=w1867, "input_error"=w1863, "input_Iexist"=w1866, "input_filePath"=w1865, "input_hdl_Workbooks"=w1864) -> ("output_error"=w1861:errorcluster, "output_newFilePath"=w1860:path, "output_hdl_Worksbooks"=w1862:refnum<k7>)  [unwired: 4 in]
            }
          }
          n199 = case shown="True" w1771 {
            selector: w1771 -> [_ w1856]
            tunnel: w1770 -> [_ w1855]
            tunnel: w1769 -> [w1848 w1854]
            tunnel: w1768 -> [w1847 w1853]
            tunnel: [w1847 w1851] -> w1719
            tunnel: [w1848 w1852] -> w1718
            tunnel: [w1846 w1850] -> w1766
            tunnel: w1767 -> [w1846 _]
            frame False {
            }
            frame True {
              n200 = call "myRIO_BRig_Host_formatData_getHeaders_dataCurrent.vi"() -> ("output_stringArray_dataCurrent"=w1849:string[])  [unwired: 11 in]
              n201 = call "myRIO_BRig_Host_formatData_test3_p2.vi"("input_headers"=w1849, "input_error"=w1853, "input_Iexist"=w1856, "input_filePath"=w1855, "input_hdl_Workbooks"=w1854) -> ("output_error"=w1851:errorcluster, "output_newFilePath"=w1850:path, "output_hdl_Worksbooks"=w1852:refnum<k7>)  [unwired: 4 in]
            }
          }
          n202 = case shown="True" w1742 {
            selector: w1742 -> [_ w1845]
            tunnel: w1729 -> [_ w1844]
            tunnel: w1718 -> [w1837 w1843]
            tunnel: w1719 -> [w1836 w1842]
            tunnel: [w1836 w1840] -> w1717
            tunnel: [w1837 w1841] -> w1716
            tunnel: [w1835 w1839] -> w1707
            tunnel: w1727 -> [w1835 _]
            frame False {
            }
            frame True {
              n203 = call "myRIO_BRig_Host_formatData_getHeaders_dataExp.vi"() -> ("output_stringArray_dataExp"=w1838:string[])  [unwired: 11 in]
              n204 = call "myRIO_BRig_Host_formatData_test3_p2.vi"("input_headers"=w1838, "input_error"=w1842, "input_Iexist"=w1845, "input_filePath"=w1844, "input_hdl_Workbooks"=w1843) -> ("output_error"=w1840:errorcluster, "output_newFilePath"=w1839:path, "output_hdl_Worksbooks"=w1841:refnum<k7>)  [unwired: 4 in]
            }
          }
          n205 = case shown="True" w1730 {
            selector: w1730 -> [_ w1834]
            tunnel: w1728 -> [_ w1833]
            tunnel: w1716 -> [w1826 w1832]
            tunnel: w1717 -> [w1825 w1831]
            tunnel: [w1825 w1829] -> w1714
            tunnel: [w1826 w1830] -> w1715
            tunnel: [w1824 w1828] -> w1706
            tunnel: w1726 -> [w1824 _]
            frame False {
            }
            frame True {
              n206 = call "myRIO_BRig_Host_formatData_getHeaders_dataLC.vi"() -> ("output_stringArray_dataLC"=w1827:string[])  [unwired: 11 in]
              n207 = call "myRIO_BRig_Host_formatData_test3_p2.vi"("input_headers"=w1827, "input_error"=w1831, "input_Iexist"=w1834, "input_filePath"=w1833, "input_hdl_Workbooks"=w1832) -> ("output_error"=w1829:errorcluster, "output_newFilePath"=w1828:path, "output_hdl_Worksbooks"=w1830:refnum<k7>)  [unwired: 4 in]
            }
          }
          n208 = case shown="True" w1731 {
            selector: w1731 -> [_ w1823]
            tunnel: w1724 -> [_ w1822]
            tunnel: w1715 -> [w1815 w1821]
            tunnel: w1714 -> [w1814 w1820]
            tunnel: [w1814 w1818] -> w1712
            tunnel: [w1815 w1819] -> w1713
            tunnel: [w1813 w1817] -> w1705
            tunnel: w1725 -> [w1813 _]
            frame False {
            }
            frame True {
              n209 = call "myRIO_BRig_Host_formatData_getHeaders_dataLick.vi"() -> ("output_stringArray_dataLick"=w1816:string[])  [unwired: 11 in]
              n210 = call "myRIO_BRig_Host_formatData_test3_p2.vi"("input_headers"=w1816, "input_error"=w1820, "input_Iexist"=w1823, "input_filePath"=w1822, "input_hdl_Workbooks"=w1821) -> ("output_error"=w1818:errorcluster, "output_newFilePath"=w1817:path, "output_hdl_Worksbooks"=w1819:refnum<k7>)  [unwired: 4 in]
            }
          }
          n211 = case shown="True" w1732 {
            selector: w1732 -> [_ w1812]
            tunnel: w1723 -> [_ w1811]
            tunnel: w1713 -> [w1804 w1810]
            tunnel: w1712 -> [w1803 w1809]
            tunnel: [w1803 w1807] -> w1710
            tunnel: [w1804 w1808] -> w1711
            tunnel: [w1802 w1806] -> w1704
            tunnel: w1722 -> [w1802 _]
            frame False {
            }
            frame True {
              n212 = call "myRIO_BRig_Host_formatData_getHeaders_dataMTrig.vi"() -> ("output_stringArray_dataMTrig"=w1805:string[])  [unwired: 11 in]
              n213 = call "myRIO_BRig_Host_formatData_test3_p2.vi"("input_headers"=w1805, "input_error"=w1809, "input_Iexist"=w1812, "input_filePath"=w1811, "input_hdl_Workbooks"=w1810) -> ("output_error"=w1807:errorcluster, "output_newFilePath"=w1806:path, "output_hdl_Worksbooks"=w1808:refnum<k7>)  [unwired: 4 in]
            }
          }
          n214 = case shown="True" w1733 {
            selector: w1733 -> [_ w1801]
            tunnel: w1721 -> [_ w1800]
            tunnel: w1711 -> [w1793 w1799]
            tunnel: w1710 -> [w1792 w1798]
            tunnel: [w1792 w1796] -> w1708
            tunnel: [w1793 w1797] -> w1709
            tunnel: [w1791 w1795] -> w1703
            tunnel: w1720 -> [w1791 _]
            frame False {
            }
            frame True {
              n215 = call "myRIO_BRig_Host_formatData_getHeaders_dataTrial.vi"() -> ("output_stringArray_dataTrial"=w1794:string[])  [unwired: 11 in]
              n216 = call "myRIO_BRig_Host_formatData_test3_p2.vi"("input_headers"=w1794, "input_error"=w1798, "input_Iexist"=w1801, "input_filePath"=w1800, "input_hdl_Workbooks"=w1799) -> ("output_error"=w1796:errorcluster, "output_newFilePath"=w1795:path, "output_hdl_Worksbooks"=w1797:refnum<k7>)  [unwired: 4 in]
            }
          }
        }
        frame #5 {
          # "Re-check\nlabel\npart2"
          n217 = Not(x=w1888) -> (.not. x?=w1893:bool)
          n218 = Not(x=w1892) -> (.not. x?=w1897:bool)
          n219 = Not(x=w1889) -> (.not. x?=w1894:bool)
          n220 = Not(x=w1891) -> (.not. x?=w1896:bool)
          n221 = Not(x=w1923) -> (.not. x?=w1924:bool)
          n222 = Not(x=w1890) -> (.not. x?=w1895:bool)
          n223 = Not(x=w1930) -> (.not. x?=w1933:bool)
          n224 = case shown="True" w1893 {
            tunnel: w1882 -> [w1942 w1947]
            tunnel: w1883 -> [_ w1946]
            tunnel: [w1942 w1945] -> w1868
            tunnel: [w1943 w1944] -> w1869
            tunnel: w1888 -> [w1943 _]
            frame False {
            }
            frame True {
              n225 = call "myRIO_BRig_generic_pathExists_fast_pathInput.vi"("input_error"=w1947, "input_filePath"=w1946) -> ("output_error"=w1945:errorcluster, "output_Iexist"=w1944:bool)  [unwired: 7 in, 1 out]
            }
          }
          n226 = case shown="True" w1897 {
            tunnel: w1878 -> [w1966 w1971]
            tunnel: w1887 -> [_ w1970]
            tunnel: [w1966 w1969] -> w1876
            tunnel: [w1967 w1968] -> w1877
            tunnel: w1892 -> [w1967 _]
            frame False {
            }
            frame True {
              n227 = call "myRIO_BRig_generic_pathExists_fast_pathInput.vi"("input_error"=w1971, "input_filePath"=w1970) -> ("output_error"=w1969:errorcluster, "output_Iexist"=w1968:bool)  [unwired: 7 in, 1 out]
            }
          }
          n228 = case shown="True" w1894 {
            tunnel: w1881 -> [w1948 w1953]
            tunnel: w1884 -> [_ w1952]
            tunnel: [w1948 w1951] -> w1870
            tunnel: [w1949 w1950] -> w1871
            tunnel: w1889 -> [w1949 _]
            frame False {
            }
            frame True {
              n229 = call "myRIO_BRig_generic_pathExists_fast_pathInput.vi"("input_error"=w1953, "input_filePath"=w1952) -> ("output_error"=w1951:errorcluster, "output_Iexist"=w1950:bool)  [unwired: 7 in, 1 out]
            }
          }
          n230 = case shown="True" w1896 {
            tunnel: w1879 -> [w1960 w1965]
            tunnel: w1886 -> [_ w1964]
            tunnel: [w1960 w1963] -> w1874
            tunnel: [w1961 w1962] -> w1875
            tunnel: w1891 -> [w1961 _]
            frame False {
            }
            frame True {
              n231 = call "myRIO_BRig_generic_pathExists_fast_pathInput.vi"("input_error"=w1965, "input_filePath"=w1964) -> ("output_error"=w1963:errorcluster, "output_Iexist"=w1962:bool)  [unwired: 7 in, 1 out]
            }
          }
          n232 = case shown="True" w1924 {
            tunnel: w1899 -> [w1972 w1977]
            tunnel: w1922 -> [_ w1976]
            tunnel: [w1972 w1975] -> w1898
            tunnel: [w1973 w1974] -> w1921
            tunnel: w1923 -> [w1973 _]
            frame False {
            }
            frame True {
              n233 = call "myRIO_BRig_generic_pathExists_fast_pathInput.vi"("input_error"=w1977, "input_filePath"=w1976) -> ("output_error"=w1975:errorcluster, "output_Iexist"=w1974:bool)  [unwired: 7 in, 1 out]
            }
          }
          n234 = case shown="True" w1895 {
            tunnel: w1880 -> [w1954 w1959]
            tunnel: w1885 -> [_ w1958]
            tunnel: [w1954 w1957] -> w1872
            tunnel: [w1955 w1956] -> w1873
            tunnel: w1890 -> [w1955 _]
            frame False {
            }
            frame True {
              n235 = call "myRIO_BRig_generic_pathExists_fast_pathInput.vi"("input_error"=w1959, "input_filePath"=w1958) -> ("output_error"=w1957:errorcluster, "output_Iexist"=w1956:bool)  [unwired: 7 in, 1 out]
            }
          }
          n236 = case shown="True" w1933 {
            tunnel: w1929 -> [w1978 w1983]
            tunnel: w1932 -> [_ w1982]
            tunnel: [w1978 w1981] -> w1900
            tunnel: [w1979 w1980] -> w1931
            tunnel: w1930 -> [w1979 _]
            frame False {
            }
            frame True {
              n237 = call "myRIO_BRig_generic_pathExists_fast_pathInput.vi"("input_error"=w1983, "input_filePath"=w1982) -> ("output_error"=w1981:errorcluster, "output_Iexist"=w1980:bool)  [unwired: 7 in, 1 out]
            }
          }
        }
      }
      n238 = Merge Errors(w925, w926, w928, w927, w923, w922, w921) -> (w924:errorcluster)
    }
  }
  "error1" <- w288
  n239 = Boolean To (0,1)(Boolean=w16) -> (0, 1=w33:i16)
  n240 = Boolean To (0,1)(Boolean=w17) -> (0, 1=w32:i16)
  n241 = Boolean To (0,1)(Boolean=w18) -> (0, 1=w31:i16)
  n242 = Boolean To (0,1)(Boolean=w284) -> (0, 1=w281:i16)
  n243 = Boolean To (0,1)(Boolean=w283) -> (0, 1=w280:i16)
  n244 = Boolean To (0,1)(Boolean=w282) -> (0, 1=w279:i16)
  n245 = Boolean To (0,1)(Boolean=w7) -> (0, 1=w51:i16)
  n246 = Boolean To (0,1)(Boolean=w8) -> (0, 1=w50:i16)
  n247 = Boolean To (0,1)(Boolean=w9) -> (0, 1=w49:i16)
  n248 = Boolean To (0,1)(Boolean=w240) -> (0, 1=w246:i16)
  n249 = Boolean To (0,1)(Boolean=w239) -> (0, 1=w245:i16)
  n250 = Boolean To (0,1)(Boolean=w238) -> (0, 1=w244:i16)
  n251 = Boolean To (0,1)(Boolean=w10) -> (0, 1=w45:i16)
  n252 = Boolean To (0,1)(Boolean=w11) -> (0, 1=w44:i16)
  n253 = Boolean To (0,1)(Boolean=w12) -> (0, 1=w43:i16)
  n254 = Boolean To (0,1)(Boolean=w13) -> (0, 1=w39:i16)
  n255 = Boolean To (0,1)(Boolean=w14) -> (0, 1=w38:i16)
  n256 = Boolean To (0,1)(Boolean=w15) -> (0, 1=w37:i16)
  n257 = Boolean To (0,1)(Boolean=w21) -> (0, 1=w27:i16)
  n258 = Boolean To (0,1)(Boolean=w20) -> (0, 1=w26:i16)
  n259 = Boolean To (0,1)(Boolean=w19) -> (0, 1=w25:i16)
  n260 = Compound Arithmetic op=ADD(w33, w32, w31) -> (w30:i16)
  n261 = case shown="3" w30 {
    tunnel: ["!!!  Error - Missing  !!!" "! Error - Saving !" "Error - Labelling" "Success"] -> w29
    frame 0, Default {
    }
    frame 1 {
    }
    frame 2 {
    }
    frame 3 {
    }
  }
  n262 = Compound Arithmetic op=ADD(w281, w280, w279) -> (w278:i16)
  n263 = case shown="3" w278 {
    tunnel: ["!!!  Error - Missing  !!!" "! Error - Saving !" "Error - Labelling" "Success"] -> w277
    frame 0, Default {
    }
    frame 1 {
    }
    frame 2 {
    }
    frame 3 {
    }
  }
  n264 = Compound Arithmetic op=ADD(w51, w50, w49) -> (w48:i16)
  n265 = case shown="3" w48 {
    tunnel: ["!!!  Error - Missing  !!!" "! Error - Saving !" "Error - Labelling" "Success"] -> w47
    frame 0, Default {
    }
    frame 1 {
    }
    frame 2 {
    }
    frame 3 {
    }
  }
  n266 = Compound Arithmetic op=ADD(w246, w245, w244) -> (w243:i16)
  n267 = case shown="3" w243 {
    tunnel: ["!!!  Error - Missing  !!!" "! Error - Saving !" "Error - Labelling" "Success"] -> w242
    frame 0, Default {
    }
    frame 1 {
    }
    frame 2 {
    }
    frame 3 {
    }
  }
  n268 = Compound Arithmetic op=ADD(w45, w44, w43) -> (w42:i16)
  n269 = case shown="3" w42 {
    tunnel: ["!!!  Error - Missing  !!!" "! Error - Saving !" "Error - Labelling" "Success"] -> w41
    frame 0, Default {
    }
    frame 1 {
    }
    frame 2 {
    }
    frame 3 {
    }
  }
  n270 = Compound Arithmetic op=ADD(w39, w38, w37) -> (w36:i16)
  n271 = case shown="3" w36 {
    tunnel: ["!!!  Error - Missing  !!!" "! Error - Saving !" "Error - Labelling" "Success"] -> w35
    frame 0, Default {
    }
    frame 1 {
    }
    frame 2 {
    }
    frame 3 {
    }
  }
  n272 = Compound Arithmetic op=ADD(w27, w26, w25) -> (w24:i16)
  n273 = case shown="3" w24 {
    tunnel: ["!!!  Error - Missing  !!!" "! Error - Saving !" "Error - Labelling" "Success"] -> w23
    frame 0, Default {
    }
    frame 1 {
    }
    frame 2 {
    }
    frame 3 {
    }
  }
  n274 = case shown="False" w293 {
    tunnel: w294 -> [w2015 w2021]
    tunnel: w296 -> [w2014 w2019]
    tunnel: [w2018 w2021] -> w289
    tunnel: [w2017 w2020] -> w291
    tunnel: w295 -> [w2013 w2020]
    tunnel: [w2012 w2019] -> w292
    frame False {
      n275 = invoke class="Workbooks" method="Close"(reference=w2014, error in=w2015) -> (reference out=w2012:refnum<k7>, error out=w2016:errorcluster)  [unwired: 1 in, 1 out]
      n276 = invoke class="_Application" method="Quit"(reference=w2013, error in=w2016) -> (reference out=w2017:refnum<k7>, error out=w2018:errorcluster)  [unwired: 1 in, 1 out]
    }
    frame True {
    }
  }
  n277 = Concatenate Strings("DataMTrig = ", w29) -> (w3:string)
  n278 = Concatenate Strings("DataBlock = ", w277) -> (w237:string)
  n279 = Concatenate Strings("DataExp = ", w47) -> (w6:string)
  n280 = Concatenate Strings("DataCurrent = ", w242) -> (w236:string)
  n281 = Concatenate Strings("DataLC = ", w41) -> (w5:string)
  n282 = Concatenate Strings("DataLick = ", w35) -> (w4:string)
  n283 = Concatenate Strings("DataTrial = ", w23) -> (w1:string)
  n284 = Concatenate Strings(w237, w2, w236, w2, w6, w2, w5, w2, w4, w2, w3, w2, w1) -> (w235:string)
  n285 = flat-sequence {
    tunnel: w235 -> [w2023]
    tunnel: [w2022] -> w53
    tunnel: w52 -> [w2022]
    frame #0 {
      n286 = One Button Dialog(message=w2023) -> ()  [unwired: 1 in, 1 out]
    }
  }
  n287 = Close Reference(reference=w292, error in (no error)=w289) -> (error out=w290:errorcluster)
  n288 = Unbundle By Name(w53) -> ("code"=w287:i32)
  n289 = Close Reference(reference=w291, error in (no error)=w290) -> (error out=w52:errorcluster)
  "error2" <- w52
  n290 = Equal?(x=w287, y=-2146827284) -> (x = y?=w285:bool)
  n291 = case shown="True" w285 {
    frame False {
    }
    frame True {
      n292 = One Button Dialog(message="Use \"Alt-Ctrl-Delete\" to close Excel") -> ()  [unwired: 1 in, 1 out]
    }
  }
